vi "Supplementary Fig.10.vi"(3 "filepath":path) -> ()   [LabVIEW 2018]
uses:
  <vilib>/Utility/miscctls.llb/LVBoundsTypeDef.ctl
  <vilib>/Utility/file.llb/Read Delimited Spreadsheet (I64).vi
  <vilib>/Analysis/3filter.llb/Butterworth Filter (DBL).vi
  <vilib>/Analysis/NI_AALBase.lvlib
panel:
  out "current file index":i32
  in  "x":dbl
  out "output variable":dbl=68.582008670742
  in  "PCOcompressed":bool
  out "appended path":path=path "D:/大学/conference paper workshop/2018ViFFI/NCommn/reportchecklist/testimages.tif"
  out "size(s)":i32[](array[numeric])=[50, 88, 2560]
  in  "go":bool
  out "Array":path[](array[path])
  in  "review all files":bool
  out "img len 2":i32=70
  out "Boolean":bool=TRUE
  out "cs 3":dbl[](graph)=[22.65040892157367, 86.37730490337717, 155.79963793803236, 197.17804143502852, 212.85393455413336, 213.6452450101584, 210.82573019637186, 209.85631744380734, 208.5153495857973, 205.32869587141286, 202.08786171253874, 200.58274723476814, 201.02503833297055, 202.13900135116626, 202.65130109889043, 201.8843012705394, 200.89276924196565, 200.89702800042315, 201.32918494553184, 201.83283790754814, 202.84705166948518, 203.83063939953993, 203.44359282126754, 202.45792601226054, 202.63395668821033, 202.93321345821835, 203.15667855475328, 204.43918408682885, 205.67148460577496, 205.62475824945588, 205.46283059740284, 205.8138945597605, 205.80833242991133, 205.58843600987532, 204.60192113663442, 203.06170729060165, 202.23131126048585, 201.8641799176052, 201.30668848010538, 201.19635084533294, 201.96157151537406, 202.71980769348514, 203.27723713412033, 203.94056554984283, 204.18488561830355, 202.82728829485137, 201.36826216771493, 201.03099802192392, 200.7112090135604, 200.91265471875832, 201.30680696006576, 201.12311332384192, 201.40432765992006, 202.3164767282985, 202.39930349464566, 201.78281933763196, 202.24792538060763, 203.3800816469132, 203.31614273423315, 201.80453332483162, 200.49831835013848, 201.0398808130734, 202.0835068642121, 203.17981933909138, 205.62291661530793, 208.24427083572772, 211.36580763125718, 217.1450167772106, 226.14185557611017, 237.09115177491964, 246.07502920376032, 250.50482038078198, 254.51794286038157, 261.0230900964432, 269.72373715173757, 281.32337460851846, 292.9717516954466, 301.74712935377573, 308.96914350623297, 314.5127261014365, 315.7698306771272, 315.2048104451725, 316.4985840808151, 319.17590958776924, 320.2925476750582, 318.79315408433484, 319.15518315897964, 321.16787818269864, 322.6518956719798, 325.82091926094574, 331.1453319723793, 339.1117692119619, 344.0667454499893, 342.5681441424036, 343.2135713055129, 346.86002753615367, 351.44963207356125, 358.4665102360143, 359.9398685334197, 351.27714990813155, 334.9058862689725, 313.08353183385304, 303.43364672805143, 320.9407183868012, 342.12763830096344, 334.0072827765716, 298.20071977469155, 256.60459772605424, 223.36742331526776, 203.4557119569053, 196.15235288354899, 196.00154810766026, 197.8056656612016, 199.75213440726253, 201.7669588058611, 203.60351698833327, 203.29659749416388, 201.41873422982093, 200.72688499277828, 200.99345091694389, 202.06117453039934, 203.4671340637097, 204.4367775526614, 205.3704683880752, 205.2441285428637, 204.0327353325124, 203.2256293614327, 202.57558707235418, 202.03649450261787, 202.3307003542739, 202.29962244985785, 201.48883579279754, 201.2229334678881, 202.2188113001841, 204.41794090834088, 206.06170983615206, 205.41396074677795, 203.66954763507547, 202.92423305479753, 202.99827691279836, 202.73073788739418, 202.5514494622047, 202.862118680771, 203.0195210914974, 203.0643651013083, 203.63996340660358, 204.55821898163626, 204.45104395499254, 203.16523352272313, 202.1839469761759, 202.46843320863397, 203.55190028100589, 203.892787651315, 204.14591687422634, 204.75909563552855, 203.8859946870238, 202.07738571462303, 200.76087754519654, 201.29410427246535, 204.96934135088196]
  in  "low cutoff freq: fl 2":dbl=0.12500000000000006 format="%0.4f"
  in  "low cutoff freq: fl":dbl=0.12500000000000006 format="%0.4f"
  out "result":bool=TRUE
  out "x < y?":bool=TRUE
  in  "Threshold Limits 2":cluster{"Lower value":sgl, "Upper value":sgl}={"Lower value"=20.0, "Upper value"=60005.0} {"Upper value" format="%.2f"; "Lower value" format="%.2f"}
  in  "Threshold Limits":cluster{"Lower value":sgl, "Upper value":sgl}={"Lower value"=50.0, "Upper value"=60000.0} {"Upper value" format="%.2f"; "Lower value" format="%.2f"}
  in  "reverse v":bool
  in  "low limit":i32=81
  in  "up limit":i32=3
  in  "h/v align":bool=TRUE
  out "img len":i32=78
  in  "v cut param":T1={"thresh"=60.0, "ch1 back"=20.0, "img len"=70, "ch2 ofst"=68, "add ofst"=0, "debris size"=0.0}
  in  "h cut param":T1={"thresh"=1500.0, "ch1 back"=7.0, "img len"=78, "ch2 ofst"=70, "add ofst"=0, "debris size"=15.0}
  out "cs 2":dbl[][](graph)
  in  "thresh2":dbl=1000.0
  out "xy shift":i32[](array[numeric])=[-1, 2]
  in  "y shift":dbl=2.0
  in  "intervals":i32=40
  out "Histogram":T2(graph)={"X Values"=[4559.940789473683, 4813.127631578946, 5066.31447368421, 5319.501315789473, 5572.688157894736, 5825.874999999999, 6079.061842105262, 6332.248684210525, 6585.435526315789, 6838.622368421052, 7091.809210526315, 7344.996052631578, 7598.182894736841, 7851.369736842104, 8104.556578947368, 8357.74342105263, 8610.930263157894, 8864.117105263158, 9117.303947368422, 9370.490789473686, 9623.67763157895, 9876.864473684214, 10130.051315789478, 10383.238157894742, 10636.425000000007, 10889.61184210527, 11142.798684210535, 11395.985526315799, 11649.172368421063, 11902.359210526327, 12155.546052631591, 12408.732894736855, 12661.91973684212, 12915.106578947383, 13168.293421052647, 13421.480263157911, 13674.667105263175, 13927.85394736844, 14181.040789473704, 14434.227631578968], "Histogram: h(x)"=[13, 6, 12, 7, 11, 10, 12, 18, 10, 17, 8, 14, 12, 14, 15, 16, 28, 30, 21, 12, 10, 11, 4, 5, 5, 7, 7, 8, 6, 2, 5, 10, 4, 4, 6, 5, 3, 3, 1, 2]}
  out "cs":dbl[][](graph)
  in  "skip failed img":bool
  in  "decline thresh":dbl=20.0
  in  "color 1":T3={"color array"=[0, 65280, 16776960, 16448250, 65280, 16776960, 16711680, 16448250, 16448250], "num of colors"=4, "max"=24.0, "min"=0.0} {"min" step=0.01 format="%_2f"; "max" step=0.1 format="%_3f"}
  in  "mgn":i32[](array[numeric])=[10, 10, 10, 10]
  in  "iter":i32=10
  in  "input 2":T4={"Niblack Dev Fac"=0.6000000000000001, "Window"={"Width"=50, "Height"=50}, "Sauvola Dev Rng"=2.0, "adaptive"=FALSE, "Method (Niblack)"=1} {"Method (Niblack)" items=["Niblack", "Background Correction", "Sauvola"]}
  in  "in1":T4={"Niblack Dev Fac"=0.5, "Window"={"Width"=20, "Height"=20}, "Sauvola Dev Rng"=6000.0, "adaptive"=FALSE, "Method (Niblack)"=0} {"Method (Niblack)" items=["Niblack", "Background Correction", "Sauvola"]}
  in  "post proc 2":T5={"trunc for ch2 masking"=[2, 2, 5, 2], "Erosion(pre)"=2, "Op"=enum."PClose", "post proc"=TRUE, "move x/y"=[0, 0], "conv"=FALSE, "Conn"=TRUE, "iterations"=5, "Erosion(post)"=2}
  in  "post proc1":T6={"trunc for ch2 masking"=[0, 0, 0, 0], "Erosion(pre)"=2, "Op"=enum."PClose", "post proc"=TRUE, "move x/y"=[0, 0], "conv"=TRUE, "Conn"=TRUE, "iteration"=5, "Erosion(post)"=2}
  in  "seg meth 2":T7={"norm for thresh"=TRUE, "use thresh formula"=FALSE, "thresh"=0.27000000000000013, "man thresh"=FALSE, "Meth"=0, "upper lim"=65000} {"Meth" items=["clustering", "entropy", "metric", "moments", "inter-class variance"]; "thresh" format="%_3g"}
  in  "seg meth":T7={"norm for thresh"=TRUE, "use thresh formula"=FALSE, "thresh"=3.378, "man thresh"=FALSE, "Meth"=0, "upper lim"=64100} {"Meth" items=["clustering", "entropy", "metric", "moments", "inter-class variance"]; "thresh" format="%_3g"}
  out "mask2":u8[][](graph)
  in  "lpf 2":cluster{"cut":dbl, "lpf":bool, "odr":i32}={"cut"=0.2900001, "lpf"=FALSE, "odr"=2} {"cut" min=1e-07 max=0.4999 step=0.01 format="%_2g"}
  in  "bg calc rng":dbl[](array[numeric])=[0.4, 0.6]
  in  "bg":u16(ring)=2 items=["calc bg", "load bg", "no bg correction"]
  out "cells":i32
  out "x = y?":bool
  in  "lpf 1":cluster{"cut":dbl, "lpf":bool, "odr":i32}={"cut"=0.15000010000000014, "lpf"=FALSE, "odr"=2} {"cut" min=1e-07 max=0.4999 step=0.01 format="%_2g"}
  out "mask1":u8[][](graph)
  in  "idx2":i32
  in  "show imgs":bool=TRUE
  out "N of success":u16=10
  in  "bg filepath":path
  in  "search subholder":bool
  in  "save img":bool
  in  "mask img":bool=TRUE
  in  "sec unit":i32=300
  in  "scale fac1":dbl=1.0000000000000009 min=0.01 max=10.0 step=0.01 format="%_3g"
  in  "scale fac2":dbl=0.9999999999999983 min=0.01 max=10.0 step=0.01 format="%_3g"
  in  "autoscale":bool=TRUE
  out "ch2":picture
  out "ch1":picture
  in  "color":T8(array[cluster])=[{"color array"=[0, 16711680, 16776960, 16448250, 65280, 16776960, 16711680, 16448250, 16448250], "num of colors"=2, "max"=4900.0, "min"=0.0}, {"color array"=[0, 65280, 16776960, 16448250, 65280, 16776960, 16711680, 16448250, 16448250], "num of colors"=2, "max"=9000.0, "min"=0.0}, {"color array"=[0, 255, 16448250, 16448250, 16776960, 16711680, 16448250, 16448250], "num of colors"=2, "max"=1.0, "min"=0.0}] {"min" step=0.01 format="%_2f"; "max" step=0.1 format="%_3f"}
  in  "unmix":T9={"c1 -> c2, c1 <- c2"=[0.03, 0.02000000000000004], "unmix"=FALSE}
  in  "image lpf":cluster{"cut":dbl, "lpf":bool, "odr":i32}={"cut"=0.2500001000000001, "lpf"=FALSE, "odr"=2} {"cut" min=1e-07 max=0.4999 step=0.01 format="%_2g"}
  in  "reverse h":bool
  out "mixed":picture
  out "curr img size":i32[](array[numeric])=[2560, 88]
  out "curr index":i32=1311
  in  "review all imgs":bool
  out "num of files":i32=50
  out "max2":dbl=17870.242105263158
  out "max1":dbl=14560.82105263158
  in  "file type":string=".tif"
  in  "frame index":i32 min=0 max=49
  in  "transpose":bool=TRUE
  in  "Draw Area Size":T10
  out "max value":dbl=24.0
  in  "autoscale":bool=TRUE
  in  "zoom 2":dbl=0.5000000000000014 format="%_2g"
  in  "frame [ms]":u32
  out "cycle time":u32=17
  in  "zoom":dbl=1.9999999999999973 format="%_2g"
  out "entire img":dbl[][](graph)
  out "x proj":dbl[](graph)=[-0.6834175105647228, -2.7922158127679118, -6.30996339498379, -10.48569202110438, -13.54291741641208, -14.349970108657555, -13.701267260419232, -13.894588588034273, -14.878874404013395, -14.863747871840786, -15.302439752050166, -16.30687103819798, -15.643161215622314, -14.487337019319579, -14.595162853469436, -14.593941392233873, -14.166323551069151, -14.251724102511528, -14.572410867893547, -15.041552545206267, -15.572230117774634, -15.818546099314855, -15.190464999042959, -14.320936985804096, -14.686809209149082, -15.419230593399906, -15.20675810543543, -13.981248077775604, -11.920339576425084, -10.971586187658659, -11.25221777963731, -11.344895546808072, -12.022146630222142, -13.117927850718345, -14.413445296549057, -15.269610451173484, -14.961554040865941, -14.580989432911498, -14.81303051441752, -15.451549032211478, -15.195154453333984, -14.838214893162156, -16.149251075164745, -16.918501257161715, -16.132803421003587, -15.52614796154118, -15.508980206767735, -15.695012778831137, -15.876128554725758, -16.18013743433353, -16.89454319413985, -17.46675511064096, -16.694164623634443, -14.993973438041495, -13.648547978181846, -12.653905866235657, -12.45751666205452, -13.775479390585971, -15.669316073200875, -16.82025936546387, -16.200158411236686, -13.572145620867065, -11.203500645851197, -11.017897885818662, -11.632458250522696, -11.980845686827687, -12.885503640350821, -14.208080630663469, -15.543989815895518, -16.460269150631753, -16.0001628738515, -15.358575144040161, -15.492835627959574, -15.540386983916306, -15.052309972922913, -14.088140737295321, -13.341805601328163, -13.447699196986228, -14.186839306825282, -14.653147274282508, -14.45588231379865, -14.11446313631473, -14.639373619143873, -16.322012163187026, -17.538186689406707, -16.952354638933542, -15.115955719718634, -15.92300531539663, -20.713119497102248, -23.007644467175748, -20.547675366789306, -17.36592152730349, -14.893231720663183, -13.13438666240775, -11.909837282538096, -10.365292012040246, -9.610157111318731, -10.877523616870858, -13.202799507317867, -15.167897285029014, -15.659730836338658, -14.784985852331703, -13.893954928165991, -14.028882088433711, -14.35547187020653, -13.739728292820661, -13.24559856604987, -13.277869669877969, -12.691956483769992, -11.640639835026786, -11.040015534270898, -11.507597906403465, -12.636802259475491, -13.545565542634765, -13.830692185755483, -13.60132892262358, -13.87582738758939, -14.796867880930424, -15.08557833270453, -14.757870440442604, -14.84082302405131, -15.321160652800952, -15.941638596870938, -16.07362505091237, -15.40545065416542, -14.438601088064821, -12.871091717770776, -11.520250753517509, -11.452586312676168, -12.620120570977653, -14.622116896115239, -15.632283681879436, -15.136297369122076, -14.33195472703209, -14.03183520127222, -14.016994012860485, -13.61488608346895, -13.14309108181286, -12.441790173190853, -12.035493409162154, -12.764879772451389, -13.197459793492103, -12.87401599608488, -13.303556575539167, -13.42582162495954, -12.519234369430755, -12.892944639653322, -14.230895323758885, -15.270126162912508, -15.803938832988939, -15.179763381627646, -14.315716492920693, -14.490192341186564, -15.333229669789583, -15.874632123623439, -16.10405880936504, -15.456479367886422, -14.086042542839127, -13.888521783534085, -13.475692190212179, -11.297322584278787, -9.771670180089135, -10.719122741028414, -12.901988966851139, -14.93709067962128, -16.42107411849932, -15.970247009387723, -13.976600186118329, -13.028296221958328, -12.994037757345598, -12.78968452385558, -13.09659330053799, -14.039853852258632, -14.826865503427738, -14.961553801260065, -14.338046564506225, -13.119515767298509, -12.666665024518577, -13.62220091151925, -14.283514741181664, -14.19797114502582, -14.58029943646456, -14.676383319724124, -13.370325361607014, -12.30219629465311, -12.413924716022782, -12.582413085396315, -12.996915855133329, -14.014967534975739, -14.54373505480318, -14.995804512257399, -15.636288135977123, -15.210772411813558, -14.107942433807814, -13.014760788061801, -12.742233532780755, -14.411783421344659, -16.3695857888955, -17.463640787256267, -17.940156015453052, -17.438947443968026, -16.807565061654586, -15.110157618550565, -11.670034796353715, -9.87113803290875, -11.6649752573667, -14.541639903820691, -16.07005316298409, -16.16164249576132, -15.543260514552726, -14.734452468049788, -13.885135037158573, -13.842148930997821, -14.865775635246669, -16.43097528689782, -16.784402185436797, -14.838523730819883, -12.690860817932032, -11.509913102805502, -11.600547921666902, -12.763065997311815, -13.828886943745289, -14.641508689410983, -14.759488950986187, -14.697478966043427, -15.380737221215163, -15.752696058094127, -15.192211950311329, -13.85637867630627, -12.5885088775801, -13.986311130425905, -17.484154311875482, -19.046814456908745, -18.280215041100195, -17.622357903220184, -17.06239523828483, -15.77743235808388, -15.143136249929485, -15.07106817712601, -14.335874126088605, -13.862011364263319, -14.44136253512707, -14.462116800645607, -13.214625250557301, -11.93392977639283, -11.337571166409074, -12.080897024719594, -13.761546151606957, -15.586457422748946, -17.03967711245096, -17.21569558063286, -16.018561164245824, -14.928850262697573, -14.983923288034408, -14.813297163825101, -14.145916271389098, -14.647520708873756, -16.123946788813186, -17.25110209410827, -17.82165228056119, -17.983853719926973, -18.04422638097217, -18.24234127109032, -17.530321903976997, -15.230888143169889, -12.616883481434947, -12.090427047136432, -14.027511215130799, -16.029297161120862, -16.6851178900205, -15.855121037384794, -14.072937007099437, -12.864605553004116, -13.002858586848216, -13.731244094423328, -14.17662604623215, -14.64663422697672, -15.527087976424205, -15.517100827951875, -13.94499632273175, -12.466131030389096, -12.865082244751546, -14.710482883628332, -16.024466334368416, -16.160012901234012, -14.873502217072105, -12.736706466556772, -12.615419101744688, -14.677799621809232, -15.783980088472472, -15.553650423082287, -15.553553147413675, -15.434975844288209, -14.346901786619798, -12.970057203096355, -12.620433471080204, -13.726063979269703, -15.177896881858572, -15.8852613477424, -16.26348880688422, -16.28666584690531, -15.20613082070219, -13.98440480236911, -14.6571949020836, -16.675060226670517, -17.572209949311954, -17.06201153404411, -16.672466239332874, -16.18237233298253, -14.580951850229942, -12.746327410477114, -12.038589093044003, -13.25207243640323, -15.217854714436147, -15.788037915720603, -14.986933523340761, -14.041583991859127, -14.003121141209725, -14.965392038911046, -15.202033181366888, -13.932810748930311, -12.5596649100939, -11.590493669035851, -11.13446553973715, -12.00388590594944, -13.756641248085415, -14.240668387154688, -12.74592674839886, -11.565852728612187, -11.830195142380187, -12.863301858501114, -13.846841146394226, -14.527393047335213, -16.01274997876434, -17.186307290045313, -16.33316266272545, -14.747100132132857, -13.438496507277772, -12.24526532342578, -11.654108455815297, -11.00634877930038, -9.8116388052108, -9.68222391524505, -10.934757774278028, -12.451689536930694, -13.75724845069177, -14.775390496833003, -15.39774879190061, -15.449870991671233, -14.803404143170503, -13.297855630290385, -10.922326954053016, -8.501089033287602, -7.205429067723376, -8.06015239248695, -10.664714947442652, -13.323567663388861, -15.450325890588493, -16.373906391926973, -15.266543081959618, -13.71938862801769, -13.117993888128822, -12.871449495240045, -12.058421542266892, -10.88591753675202, -11.223052351972944, -13.200944720691913, -14.953341257456014, -14.87227729819865, -13.625930847916097, -13.356565121838807, -14.591995298877666, -16.822869344770503, -18.31908536098044, -18.205058083756246, -17.69644453667013, -17.15729710527646, -16.135104370676746, -14.081883680529572, -11.998664196339602, -11.597672584201458, -11.816389488471224, -11.668106269387222, -12.138815385528066, -13.998866957004868, -16.279054868253226, -17.6135573111164, -17.818782424364908, -17.17691207732298, -15.91755610189869, -15.237073902859034, -16.479760552177495, -18.26872845243941, -18.271950732608648, -16.116568927060992, -13.692857087588177, -12.809637763557653, -13.468252056217336, -14.676499226409021, -15.010321047751553, -14.336515784833214, -13.492341077302898, -12.921047284674534, -12.956711119575031, -12.985504423910527, -13.098394139546045, -13.195229816037006, -12.760742097479472, -12.611717807950198, -12.713676672823652, -12.761848102734396, -13.066171492922482, -14.215712849893492, -15.686225069544669, -15.517883958411224, -13.599795748689289, -11.749887472784824, -10.938033179552045, -11.667925359853475, -13.798265279819777, -15.563471624573406, -16.12708652825845, -16.26532778638087, -15.817266968145418, -14.958226466408965, -15.273979649743305, -16.24854573156266, -16.378706873444983, -16.078937541330014, -15.948187403204532, -15.729575955621078, -15.469419412683399, -15.589905173116293, -15.497325866266758, -14.100675390369688, -13.01002260858952, -14.009392630337985, -15.608051868802011, -16.196372475024862, -15.437111465596924, -14.329904306370954, -13.831999607704418, -13.829270681968556, -14.773714642502364, -15.762685662610984, -15.696864318156036, -15.988567863336673, -17.06657763484871, -17.1070208228435, -15.711872633335386, -14.968819680882266, -14.53804988956229, -12.915134458882505, -11.626256120492368, -11.537848217412378, -12.17701577865142, -13.394884473127112, -14.622939454805643, -14.691387053035436, -13.370257677583378, -12.590024455920004, -13.368731780793084, -14.5582439738597, -14.443846986885811, -13.060808752441186, -12.966573004398207, -15.193729819736445, -17.22729424533496, -16.742443327373227, -14.924049179001983, -13.078374488598115, -11.944387085456592, -12.662051280789695, -14.497715957519178, -15.891544740670364, -16.007984456639228, -15.457893133394554, -15.486235259114254, -15.891582391790967, -16.0690378123424, -16.198859749361624, -16.066843092652928, -14.825160813746137, -12.722186357278648, -11.543901410225176, -11.036364121134463, -10.560090733306247, -11.93996321330335, -14.571250134871434, -15.322889793998462, -14.373398236609846, -15.277914990049853, -17.814033770381194, -18.14624458964294, -16.344879078785553, -14.633429521139025, -14.30373208482877, -15.149159984398118, -14.884563322300771, -13.962765605295242, -13.962933854061045, -13.098785510933382, -10.917167535713078, -9.538892122857916, -9.84532725000828, -10.984186487913647, -12.443923596805718, -13.733450414247018, -13.77923141023114, -12.611503291194628, -11.300036184587048, -10.940971209774544, -11.625383644835313, -12.976128639346207, -13.728592535875752, -14.280667188297699, -15.721919738640011, -16.018041133724946, -15.035760962133606, -14.596737640922434, -15.486559937461113, -16.66709569698512, -15.628517666977206, -13.279514260677752, -12.582618162434674, -13.587259011841349, -14.571480041743369, -14.774007952763377, -14.832141567687396, -14.62417901590864, -14.115838951326356, -14.779833995148683, -16.649243016540137, -18.28803813598679, -18.136030849121834, -15.493830506107296, -11.97946742634762, -10.132614024646431, -10.83204224715748, -13.083398029223806, -15.070484948474796, -15.900583316185184, -16.606631693874956, -16.89796995931394, -16.058617194458368, -15.658310428218389, -16.048837209241803, -16.6480960510551, -17.375800330503644, -17.764502484556782, -18.278930588482257, -18.243846379671464, -16.672457614616626, -15.495526034166168, -15.886011283190463, -16.25595054164054, -15.986415504979586, -15.511351276304644, -15.055670365460198, -14.979667171406987, -14.7670110909992, -14.396589267785435, -14.41113080260957, -15.231732144756222, -17.26975927958338, -18.917695908572455, -18.034683771181193, -14.993131494616081, -12.810390178707678, -13.816585221183711, -16.273864026963835, -17.47416177174676, -16.908040746418262, -15.778935330972239, -14.805480471895468, -13.77591153631215, -13.422602806751218, -13.237427641370106, -12.301932741252294, -12.16508225675907, -13.617093964198205, -15.32457377743269, -15.669348697686765, -14.644197088565672, -14.148536346702784, -14.70635763132227, -15.202234683460434, -14.995656258833773, -14.147444536898169, -13.709495549970399, -13.872223744801845, -13.585841916224943, -13.359226880225172, -14.510236733043408, -16.256744012190637, -16.836279404655404, -16.800501519538916, -16.768853487683117, -16.262786034117607, -15.405686115446294, -14.278138349083143, -13.500776093030744, -13.827138695459016, -14.589219205755747, -14.515510556569495, -13.899097320094867, -13.63540011593793, -13.982779378195001, -14.788715047312664, -15.23750324979562, -15.391979601812698, -15.680918454524143, -15.804209427048, -15.824136319785122, -15.216040145960125, -13.85503069404488, -12.969819547584507, -13.174690729924428, -13.858177661023209, -15.020071362979913, -16.66873485701156, -16.664238929804828, -15.036503828657484, -14.577300902713514, -15.663249328639887, -16.44963467352514, -16.340907713519364, -15.390484066640202, -13.651978722590698, -11.939183755923876, -11.880157685702155, -13.85990512263093, -15.160317825329965, -14.750132137535013, -13.44177909676561, -12.14971843706951, -11.953456082718917, -11.90621182826691, -12.024721375728102, -13.323774208659461, -14.801923001366326, -15.860148509894666, -16.560398969007977, -16.67259745118025, -16.349700229043975, -16.20313246033038, -16.07494837722363, -16.19821333346385, -17.33346740579777, -17.386396161562132, -15.886306971691344, -15.528308204029525, -16.08133775071093, -15.15997476313304, -13.521175788011508, -14.919261262111878, -18.44338345298166, -19.054414549237087, -16.698433481637196, -14.566409416036164, -13.927431310277164, -14.32856488214173, -14.72448779662178, -15.354580601292845, -17.085867437937466, -18.898633677958944, -19.05431973773286, -16.937118309252604, -13.61990235818136, -11.686290340813652, -12.14057497353854, -12.72526060715683, -12.344030714604456, -12.473126024343344, -13.307701318068705, -14.344407899774469, -15.141263546836994, -14.375404519900869, -12.509047499267052, -11.688133078270088, -11.82917976548044, -12.528691216613334, -14.11749210440634, -15.382257462980228, -15.166409726152107, -13.565007346029395, -11.24846029200768, -9.402937431724318, -9.11856165450807, -10.246672470805326, -11.990843911682553, -13.259227577445067, -14.068942831304195, -14.89771050318441, -14.725757562419561, -13.701596446886196, -13.67200539048654, -15.938115172230452, -18.475011940893992, -18.158829765945974, -16.52694273170763, -15.777196449867914, -14.930873710638284, -13.601819823773459, -12.82614552810636, -12.928375042868169, -13.673840344009115, -14.733119556941165, -14.409387340423788, -12.286610514595193, -10.783672360533515, -11.1482227575377, -12.285796771446254, -13.334426111164465, -14.04152306888732, -13.968113068912926, -13.565571398349089, -13.698676836408511, -14.739398987251828, -15.96912598030195, -15.610043449158876, -14.178170683874919, -13.436037636106873, -13.116007737437805, -13.549813702674452, -14.260748667757124, -14.005374008899139, -14.01578151453176, -14.598874055917594, -14.168839078092839, -12.88561652177645, -12.893069488243555, -14.20651672096117, -14.954206960763488, -14.635533897285665, -13.69533168004474, -12.426969518518016, -11.349284797834724, -11.244176651064338, -11.992463344862138, -13.709301583771888, -16.0548340297954, -17.010526303695826, -16.446299961260035, -15.40051602693702, -14.212092633843344, -13.440230958381331, -13.694440360563197, -14.972447092051977, -15.79973370749493, -15.079762962368783, -13.929943683165988, -13.866922502426146, -14.483671875294496, -14.59800045598237, -14.109683059525423, -14.001707767839312, -14.64846658968274, -14.513179835032515, -12.803208964464737, -11.333759624672707, -11.20175730172397, -11.762382910611045, -12.725470869679743, -13.837127994117441, -14.2712858436734, -13.138488539642207, -11.632864497123043, -12.153044804961448, -13.731136620911064, -13.971640615172891, -13.47709720430737, -13.223562425814698, -13.051744274980328, -13.071895234634479, -13.441059677351213, -14.270549629912857, -14.734283296974901, -14.406843575624034, -14.13881470261628, -13.799999085647505, -12.886486105644666, -11.942894201609375, -11.162509403713246, -10.546024049146379, -10.420186494698825, -10.60467190172187, -11.308707627674748, -12.594401250590288, -14.060041612350918, -15.40382034790587, -15.986938156543614, -15.600625288960723, -14.74914020283138, -13.879861174841682, -12.855970044949355, -11.301716249647402, -10.275279834758745, -10.899572702942617, -12.02556928116676, -12.586178194365536, -12.641762080841636, -12.507297433844652, -12.850150351413143, -13.315847803966317, -13.445365121143386, -13.607504880510621, -14.01009249139642, -15.11665772801527, -16.22100371378028, -15.819394213005449, -14.291589232398803, -12.887399643562539, -12.365678548794644, -12.146596233866502, -11.723426186339548, -11.788009369465076, -12.575742098585861, -13.980313420807267, -14.94434731363307, -15.092163524626866, -15.20307457271574, -15.258370441334009, -15.078271390990851, -14.499516129989622, -13.623369162084257, -12.794986153446477, -12.208397079373798, -12.614900776755476, -14.36525870469483, -16.075272898575975, -16.908774953278694, -17.710389932962833, -17.5049082548777, -15.579507183604274, -13.83271553763094, -12.437100645387138, -11.215410823715128, -10.724057723790883, -10.570404446192448, -10.686954186383158, -10.945687167366295, -11.443666266609224, -12.998494012153783, -14.78656200036396, -15.27067524086572, -14.350030334921108, -12.734880475715897, -11.909508512013375, -12.548403304808385, -13.621145225851697, -13.73615356679905, -12.51069310077562, -11.121719633782611, -10.80645615021873, -11.362738334849654, -11.699400817231883, -12.319537219395425, -13.57303518241118, -13.962345823865713, -13.325772324647668, -13.083990224824273, -14.04453777080227, -14.542589350605166, -13.910925784389027, -13.93041905315739, -15.233293807590229, -18.50541068155657, -21.741886908261225, -21.26178350956289, -18.461108327282645, -16.078271982064933, -14.277115360587644, -12.396936664914513, -11.322303804274165, -12.205060406963916, -12.809755829415959, -12.499829502583541, -13.56816018560935, -14.581069715638614, -13.617842584174491, -11.493387169082851, -9.616244959908883, -9.140396555421791, -9.024583228160164, -8.781116292097778, -9.664119708188412, -10.870672176794095, -11.713886281308476, -13.278264882086075, -15.25315238668777, -15.324430700349527, -12.78071524531497, -10.35871787720911, -9.801821667989485, -10.084107342749734, -9.364308023708855, -8.103424127983331, -9.009574882873586, -11.358138441845028, -12.098762273089559, -11.330757087376178, -11.336110973267026, -12.475840050303999, -13.2557090816447, -12.732387306856545, -11.39325202452236, -10.305143764032195, -10.018537104080119, -10.79444201776111, -11.91440095791831, -11.73536267229401, -10.31456445465864, -9.034702477349768, -8.204005366106507, -8.237961569664487, -9.523185551856013, -11.114111899956233, -12.771430088999317, -14.291811244396557, -14.68464558331928, -14.157695339682519, -13.23704388706355, -12.642326527538795, -12.876660806021794, -12.80767703768067, -12.176371726316166, -11.604165960209976, -10.786964929378746, -10.20723566408961, -10.811741671156058, -11.574918488738684, -11.800053271512475, -11.855551180696493, -12.32098554836191, -13.619981631838915, -14.884804240974551, -15.741922811310529, -14.956841537498823, -13.052273967620033, -12.299372783874109, -12.126755524109058, -12.410239617993726, -13.516098654943779, -14.464217855733967, -15.380017823504435, -16.317926871553535, -15.432463252245098, -13.308693067241252, -12.675479676662686, -13.665083418216021, -14.223375465901892, -13.150666394260757, -12.050840306239586, -12.543056892086254, -13.17846968977057, -13.222946133530801, -13.834123244453131, -14.590783215260934, -14.41702586293625, -13.122306213413552, -11.178503355468614, -9.582179516577003, -9.799027056274646, -11.609522625959602, -13.048929559694665, -13.509623689294225, -13.268905822963811, -13.08365227812627, -13.477388214534201, -13.812726124050073, -14.192902570866526, -15.415867788527835, -16.53979604394496, -16.0202178174342, -13.984139140611163, -11.944805278086763, -11.188951130657719, -11.839520471083837, -13.1929898745791, -13.373516962450047, -11.920990190059694, -10.686621265828707, -10.007022674212594, -9.09432977490276, -8.753260739931191, -9.907501611646746, -11.988099676427948, -13.272066167749838, -12.715126894280122, -11.957312827075732, -12.502427099483256, -13.171339380334809, -13.229766877526488, -13.257144235747598, -13.654004315967132, -14.019041801767395, -13.840391458738482, -13.647910211053484, -13.330725118868406, -12.90057841612064, -13.479440236065384, -14.754365065612097, -15.470528563451174, -15.623127968344837, -15.137754609320996, -14.43401160371674, -14.420462819446609, -14.739900977940186, -14.947955350479816, -15.037631507886339, -14.564672177701244, -13.79597657361985, -14.107576174369582, -15.341004473901641, -16.302394220322597, -15.723716596905879, -14.076622269077852, -13.888192260855774, -14.942987698572681, -14.731064428820757, -12.227041315981689, -10.132128920659497, -10.944322402730103, -12.310738819976537, -12.742490974405536, -13.182234034930673, -13.452910383557073, -13.171001180458148, -12.326833820640067, -11.62491493556143, -11.439790730067081, -11.499226917004197, -12.007496251695056, -12.173991894874673, -11.28286272464446, -10.191937392131718, -9.16755296287774, -8.467764765487638, -8.83287711277855, -9.605633213336676, -10.798276973743842, -13.03196194871889, -14.545090273160012, -14.250808950813825, -13.761874970003525, -13.984783803901166, -13.674504750987088, -12.526619326351087, -12.3288575037779, -13.013189708943907, -12.943256323442064, -12.844473906102783, -14.043856026578217, -14.81704751476948, -14.365176817049477, -14.169573906238394, -14.23341235221042, -14.65169400535721, -15.122405320819038, -14.352827184979844, -12.98220282379709, -11.946491828741078, -11.133995706383782, -11.10372830607823, -12.029441478755459, -12.814670288364535, -12.367740395775261, -11.684627915552433, -11.775346361270799, -11.698056400455352, -11.497316171731086, -11.236188716414595, -10.568753435422558, -10.80758048644044, -12.426800091765632, -14.361961323656292, -15.744340034497975, -16.012081146255248, -15.510823764795893, -14.85135566320602, -14.20142682233628, -13.515597516495845, -13.183265465861929, -13.68433600995715, -14.365158272549689, -14.449495850982615, -14.497331474152436, -14.319056660166714, -13.256352689490981, -12.606743934221438, -12.44615265609217, -11.632602342388832, -11.212003395703942, -12.160584146106642, -13.390376449027604, -14.62416645977322, -16.158512653180033, -16.412796196823255, -14.481360049817107, -12.087468041277797, -10.474297060057935, -9.751348876192479, -10.29088796282014, -11.040553019934777, -11.274604432917918, -11.538275087715387, -12.00174224621071, -12.643706274264076, -12.606311346762372, -12.161804915777699, -12.829127011753872, -15.168550294821006, -17.83515653009029, -18.690769581578547, -17.046483390522447, -13.356040766331608, -10.815277781574618, -11.89548568599545, -13.956098605866455, -14.757745212945501, -14.924304981900693, -14.716492429404633, -13.488734223593863, -11.619414953608375, -10.852043017159641, -11.142188532299201, -11.57389991989236, -12.567623658320665, -13.262980514943395, -13.19680370859935, -13.390781363050003, -14.572034914357149, -16.206858662407132, -16.57338550619015, -15.983484787390047, -15.402776514413032, -15.051913077062165, -15.305209572044149, -15.465712130955527, -15.044447865011149, -14.984299544964172, -15.263274732845003, -14.47240270005577, -13.438507521638453, -14.094200831437695, -15.740443649125117, -16.585816460991513, -15.662521110377188, -13.43629716616253, -12.328575730406634, -13.002591322671435, -13.22625121230874, -12.529030403845049, -12.968703900354367, -14.787211859615727, -15.183586898372699, -13.48665745494916, -12.242807384532732, -12.612048168957653, -13.374788409173135, -13.97082654255179, -14.864316374717294, -15.80092050806514, -15.995605117562182, -14.695381274616441, -12.818837171947369, -12.264070956174587, -12.659440271682886, -12.338440452592124, -11.51348485721978, -11.623757786198478, -12.197971445014415, -12.214432266664012, -12.917226781648836, -14.941175885330384, -16.51747748871717, -16.157406316169542, -14.413814434842632, -12.88996396848108, -11.839199118676369, -10.282536870841728, -8.969894432953037, -9.129890346532497, -10.30406985739453, -10.088560997290877, -8.224780176965137, -7.808631002927639, -8.52569743712918, -9.633363764868689, -11.317339105424008, -12.340522027178661, -12.353338731731588, -11.92673038981134, -12.203665463548345, -12.606965135638873, -12.016208365266875, -11.81295968144325, -12.794564637480189, -15.154615247697567, -18.41932567071891, -19.734329909573326, -18.90958025863206, -17.986557303211626, -16.414928736189026, -13.678760264659855, -11.525321006480095, -10.992881598173739, -10.818181704236554, -9.561748919246305, -8.8259303191477, -10.113101985345642, -11.864825155818297, -13.184939450160552, -13.552754200483818, -12.48318444522358, -11.44981056552491, -11.417846017790584, -11.341643221324869, -10.694666947441025, -10.891141382392043, -12.463610889318682, -14.075920025619835, -15.169494227778864, -15.663089494448236, -15.080513330128499, -13.390412770063019, -11.503007370934535, -10.67743564061183, -11.211631792396581, -13.162040206305637, -15.994410385042386, -17.428872023066205, -15.786919500591262, -13.077300426647412, -12.046275301359756, -11.977421849121562, -14.892220202890876, -20.98272607584496, -23.410164878910667, -20.7396753178756, -16.729349836027936, -14.32669726375579, -14.374540584831275, -15.122900818340119, -15.421989547409622, -14.575840037801667, -12.897337803087348, -12.2802980669837, -12.550941388487995, -12.914155198142778, -13.849799531976064, -14.610862199734187, -14.82125537362038, -15.156452696079324, -15.304717631507835, -14.649353201795044, -13.78678590091208, -13.387266606446483, -12.614701126400764, -12.01949250475467, -12.496894844823583, -12.36434837789248, -11.299199673581235, -10.339150000170875, -9.593793909939794, -10.28502380899112, -13.430688315275397, -16.361301433109183, -16.220764756735257, -14.427976957733367, -13.467983480552416, -13.746275321033943, -14.035755991351973, -13.727761673174783, -13.73141258022002, -12.958839804677618, -10.569505997658114, -9.160131177183473, -10.092270549868978, -12.026678022903294, -13.832634973168908, -14.49998073182459, -13.257970748666441, -11.57165070177774, -11.274455898729723, -12.825568581792716, -14.972823015873363, -14.918139182875695, -12.002947688038262, -8.686920295468049, -7.703843061152014, -9.932583951949606, -12.849708791265005, -13.880776105551147, -13.587607526687938, -12.576992143314625, -12.50294626543195, -14.234473030797316, -14.817712277903357, -13.130691685082429, -11.345740334467045, -11.299154062245716, -12.43600232474721, -13.42573083000977, -14.175168538524614, -14.551835684460766, -14.559517232873514, -14.63646589673399, -14.70645327662172, -14.453895237742902, -14.485345327347925, -15.575493498523887, -16.7880738336467, -16.689243157079414, -15.313191600144808, -14.048781309439551, -13.315367707404764, -12.264320245586308, -11.420223323192438, -11.951060996105562, -12.732905194538397, -12.316778353580135, -12.93303942086039, -15.312493113996211, -15.788346047145328, -13.784105023993487, -11.931132967348846, -10.754583426658161, -9.481930650538102, -8.674245286647826, -8.53223196073423, -8.66756896766784, -9.330659061459125, -10.398869426313595, -11.868375295911028, -13.190661813620695, -13.361703770586715, -13.179832574472094, -14.122921655970357, -15.072698301062449, -15.263268990621395, -15.02871747182958, -14.158270178382633, -14.001574877124392, -15.120300957518523, -16.32490886119167, -15.916142515617405, -14.250538284784126, -13.597495588284467, -13.732264585638854, -12.319647600822021, -9.868954733810195, -9.88428205474159, -12.375358653779111, -14.32833479589678, -14.362948764955359, -13.646960007638455, -12.862750270944963, -11.776266722172377, -11.892003110864275, -12.949068045114153, -13.22368211586893, -13.130235766638899, -13.341119971848332, -13.571092290323312, -13.131831098798397, -11.859985652818395, -11.29545402871754, -11.870574501814303, -12.600980491882503, -13.781324549543633, -14.943588154741594, -14.962515260638897, -13.518996903161211, -12.151725708742456, -12.613026798367272, -14.089489138990361, -15.132482007534652, -14.744991344322433, -13.934366281064744, -14.373206998812428, -15.252420495614174, -15.544546398879342, -15.624525249095306, -15.212030439374594, -14.01541840292304, -13.220002171473128, -13.259471527209476, -13.56182233647976, -13.443200669526052, -12.64479304867756, -11.736325534649179, -11.73173645968271, -13.006543072366126, -14.209971964728146, -14.23622255722228, -13.566935670238514, -12.927175744279861, -12.449468857700943, -12.505229013274658, -13.498084404471761, -14.220308579875681, -13.008179098424861, -11.429368926067909, -11.711730602241094, -12.016058436296666, -10.939656962933324, -10.311528674811338, -10.956803793057944, -11.384026813138167, -11.083569468470508, -11.243674331574933, -12.763979040525221, -15.022647434822222, -16.157216817895225, -16.0834853340417, -15.14762546536858, -13.508816897311728, -12.3733177244211, -12.825339089574651, -14.508688300366924, -16.140353513933025, -17.117585826520646, -16.421099079716377, -14.071865952161918, -11.308101384151682, -9.680739015687942, -9.751119427338061, -10.65282205742676, -11.577126385613825, -11.757477028287855, -11.912305020940494, -12.193423517287698, -11.918699881826493, -11.95650608067958, -12.767142162504575, -13.909339415348747, -14.716001285325426, -14.607641607535122, -13.748436468890192, -12.779227842323113, -12.151850898897981, -11.590530567532223, -11.075176185829488, -11.069295411076588, -12.114215413809315, -13.394228917180104, -13.471681970425102, -14.28960711678617, -17.768606697956606, -20.873628316228434, -20.591151713491897, -18.21588120998991, -15.582458205974813, -13.598506803166394, -13.38687573404677, -14.532082693435306, -14.998920348371339, -14.471537019639582, -13.623440551410654, -13.194904121816828, -13.952254580531806, -14.418612625434617, -13.72716939743817, -13.505604226335066, -13.917715947469471, -13.013278640201854, -11.63267210390307, -12.194600048040904, -13.868010483822658, -15.551300877056317, -16.775780946686954, -15.904668935759936, -14.089430194790094, -14.132843461549953, -15.364639899925951, -15.632837974055114, -14.694050146984445, -13.621922064514168, -13.509825727944278, -13.956778461663689, -13.927379621008377, -14.23883324834247, -15.030429522467443, -15.184780406528018, -14.480651953261287, -13.37481869464809, -13.152725021994561, -14.092992769045587, -14.370099416126408, -13.634517975561634, -12.848636260216932, -13.036311197462242, -14.256261980459573, -14.855728931850381, -15.209523678627798, -16.22194190406387, -16.86326523273269, -16.154127194388963, -14.588353486654398, -13.348507224045356, -12.994386745544126, -13.269062990015785, -13.157915031622792, -12.180516399836732, -10.026861503831599, -7.052971791167542, -5.845726303175387, -7.065655933704698, -8.911125000939101, -11.513610661502906, -16.085771359384218, -20.407630241165297, -21.396167138384726, -20.106500452257777, -17.975292303250065, -14.052713135740255, -9.893299871372655, -8.646128848349901, -9.149649038380884, -9.942465027564314, -11.303147630636158, -12.712263786892503, -13.29433715314628, -13.080522581482215, -13.465960398179956, -14.193519399431707, -13.677047529547702, -12.459438149125262, -12.06940874373609, -12.107555287326452, -11.785374630635854, -11.761797498768441, -11.651700172023837, -10.77470987736827, -10.277467825915608, -10.979673278610102, -12.881408081258911, -15.123729874220714, -16.213375242127398, -15.516951420075724, -13.911355183609802, -13.215512246383728, -13.485188270885878, -13.09270925438608, -12.242260189080177, -12.15706189736493, -12.653112418190535, -13.637348129567245, -14.399944283692626, -13.52164431422721, -11.75595893318745, -11.06743895840709, -11.787906478056772, -13.282462865635717, -15.037174738743053, -15.998085349678094, -15.538088020614815, -14.295939478002916, -13.180531971123715, -12.738227348669096, -13.181176418467498, -13.648596607647516, -13.258217387726916, -12.539095453937708, -12.088858272339287, -12.685126481437479, -14.276052257156362, -14.893817882725962, -14.36015787055838, -14.041620802517395, -14.407343210100926, -15.444115062987073, -16.00679225193796, -15.508281264979395, -14.75309046322542, -13.81673578444708, -13.283293467356337, -13.483001745651414, -13.360947257114628, -13.179303755658113, -13.634519887279453, -13.831356387051446, -13.474672616458133, -13.170406838904325, -12.807174757104738, -12.85903141085613, -13.028999693478996, -12.879068557054092, -12.778687104748215, -11.66008180706607, -10.346017883738256, -10.749178916360336, -11.76256623678157, -11.80256137072276, -11.307211225272418, -11.607907501581659, -12.154154457744, -11.787880351344914, -11.06520934753805, -10.994115324548536, -12.046657227914226, -13.941380915154921, -15.669789456476709, -16.374880875555537, -16.463511260164392, -16.312042315106236, -16.13969256265023, -16.613475743699894, -17.410505946841823, -17.41823906413456, -16.08591138034113, -14.339047723257266, -13.624353465567717, -13.435190070208034, -12.714027946453875, -12.097164240851823, -12.732277665749287, -14.903524601502898, -16.73889136907293, -16.67160097125667, -15.801107907384864, -14.807567162861844, -13.770488028618026, -12.44048318162648, -10.458293828966823, -9.716220244713512, -11.434675657060875, -14.278519548173552, -15.996378519028774, -15.886994941707165, -15.50414067786948, -15.472536627569049, -15.570358131141086, -15.77075088554125, -15.829444745462096, -15.622722116605129, -15.603519678921186, -15.947216208818126, -15.9847639985132, -15.124550300660953, -14.496279264610392, -15.655143644609138, -17.25004835753632, -17.391140085301487, -16.1138480811815, -13.788633252718995, -11.436377252570274, -10.28661385581536, -10.865371519497984, -13.64927432910638, -16.373937066476795, -16.159815741510023, -14.073408578500842, -12.958747399285668, -13.579614544935648, -14.634158502818572, -15.616698511715299, -15.508113952626893, -13.613760018175968, -12.449727291475458, -13.741077336409152, -15.444215816458026, -15.740820503096185, -15.843273548502562, -16.42678541479684, -15.771201787820232, -14.763345515486463, -15.105599187289858, -15.178444696731772, -14.840146325591009, -15.277962309548917, -15.901136374424986, -16.440362928888103, -16.936288057480688, -16.93121534903103, -15.784813648063682, -13.631724859607168, -11.886276109906028, -11.153609655764162, -11.43518563998699, -12.237773393998713, -13.095863869612034, -13.930243295991936, -14.13798038594174, -13.66518602540712, -12.857292312022686, -11.86267664283347, -11.487135120297612, -12.44092046313589, -13.758231634417674, -13.901227486163899, -13.108786179649282, -13.192679723469151, -14.121708854911326, -14.676748186508062, -15.085630055499376, -18.21504665612564, -23.469971789188087, -23.96413629777715, -19.261309800659447, -14.760352028259971, -12.572572541724341, -11.717340299483824, -11.737910510629993, -13.311585653957652, -14.788404070551195, -14.875154861878734, -14.952826851464643, -15.87581943152175, -16.42724129930399, -15.956045118058066, -15.523251954635352, -15.272276040774159, -15.375180213649712, -16.532168565585213, -17.295793035023163, -16.849033721701527, -15.978021366002611, -14.329432083449014, -12.772571435088384, -12.63532748368441, -13.415410486603104, -14.587152070491934, -15.431852962540443, -14.763722270717276, -13.559342430678292, -13.427601042100644, -13.997747235292175, -14.188675725698022, -13.397587518181886, -12.295206354497989, -11.714829641154736, -11.339843470310033, -10.593975584790256, -10.699177499342806, -12.609082611086368, -14.960477551778053, -16.247865706131183, -16.287304292765796, -15.700095818172116, -14.05938236117072, -12.02482152689761, -11.922727610554938, -12.992814852583335, -12.961792282780886, -12.185323884383957, -11.756496533286857, -11.51338595592265, -11.720014774658594, -12.874542808776022, -14.089428151065551, -14.557097139409045, -14.690688982261467, -15.051275208554447, -14.760922111062376, -12.804882009726088, -10.959863009382014, -11.336841875146279, -12.795422656411292, -13.849664037068719, -14.845574113696582, -15.33548227205372, -14.489091358376854, -13.430172559859205, -13.885517522128316, -14.86305594830933, -14.461333485663175, -13.659108700675612, -13.91535106399719, -14.033822650884375, -13.083793883686823, -12.636763007936601, -13.117760949772366, -13.817891523172047, -14.415279383720529, -13.96407661867457, -12.558500701850381, -11.578974086396155, -11.80741035304842, -12.739815294242774, -13.54274968099918, -13.305544323000762, -11.935580514742318, -10.723034702342199, -10.134121222769533, -10.666487717550297, -12.536285030709651, -14.121691345221883, -14.407374544445288, -13.855357257383675, -13.044420489082281, -12.366236661192442, -12.09478214544145, -12.650700087203319, -13.948726898222487, -14.791950185404366, -14.177962391580756, -12.829859354393124, -11.861149292827399, -11.5924705130499, -12.638371813427852, -14.10454090103706, -14.55243816890359, -14.388365660607171, -13.986746454083598, -13.955680289812419, -14.743681408656194, -15.985126741058364, -16.99053665840021, -16.841213597600923, -15.68187631608398, -14.540985925488581, -15.218624931416239, -17.409378785252464, -17.979757709695825, -16.029905519296086, -13.806178790415201, -13.335890583930016, -13.926634072480121, -14.152199745546865, -14.167950605401366, -13.91234995492033, -13.47085491811875, -13.725596060062536, -13.722409032465995, -14.122645924740036, -16.35604561390142, -17.54725415338212, -16.46140367769323, -14.259535934744788, -11.666865620447712, -10.63984603116789, -11.316834698114544, -12.395076670391527, -14.06466971832568, -15.66988744067283, -15.650459477653264, -14.023128242027186, -12.202448408289744, -11.02833874442465, -10.430639742498427, -10.746648971981926, -12.024866914906966, -13.515170230532556, -13.224965075370783, -10.990123165228077, -10.639557297502495, -12.811347244002373, -13.999475001843168, -13.321780810007471, -12.579695231383651, -12.88699688567723, -13.424085523379613, -13.242237224744981, -12.891759458695137, -13.11009731622383, -13.823298436189425, -14.42293161471654, -15.629217146849658, -17.152422764725593, -15.648011719686652, -11.281127354763935, -8.446508223820306, -8.69409789343333, -10.653449299697224, -12.711106850101796, -13.705074638868076, -13.9563106070234, -14.350010917804523, -14.539818734826374, -14.197013532199218, -14.201068707071617, -14.807315728171318, -15.572801322014476, -15.7995325019106, -16.051028062524303, -16.60308758277455, -15.965800634104038, -13.03305729209984, -8.918372168503772, -7.5786881117206715, -10.030329328495204, -13.666999843086876, -16.76662731126304, -17.890974171304848, -16.550974379638504, -14.327041736029882, -12.774595601926109, -13.028556960705, -14.761786800053638, -17.385179579787724, -20.061843315861786, -19.270185004150434, -15.386066467097555, -12.280863714504841, -11.33137417299727, -11.959409797262982, -12.379868611403102, -11.785887191396167, -11.378616418848623, -12.071311315228021, -12.860147250774784, -13.4706016772778, -14.759509047587892, -15.771217761243667, -15.319119364444152, -13.774592086869017, -12.46909727020089, -12.53415596266858, -13.323552043863451, -14.046115575780863, -14.366591906787292, -13.939730013944978, -13.33282424525978, -12.805284223831354, -12.217323425913849, -11.838835343350897, -12.166135654307745, -13.381928624480668, -14.90724449048842, -16.135323902713765, -16.784729654338022, -16.597111172798378, -16.39901633403579, -16.860576660433132, -17.166509376441343, -16.910567773325923, -15.88386863322424, -14.317783758092258, -13.476391043446926, -13.790933113895594, -14.270319387149836, -14.617441743168042, -14.784916414539193, -13.557901648746201, -11.857080778255735, -11.345953915941568, -11.821523470671059, -12.440270367542567, -12.47458305970277, -12.691208702239866, -13.372163117298053, -13.649071330394316, -13.487895946494772, -13.243635599575072, -13.067069863965717, -12.493866842950446, -12.207563243153844, -13.007380950740231, -13.563997631522197, -14.40796140595694, -16.189692064921566, -16.709522925272108, -15.33650999265748, -13.57585081331567, -12.66644961623942, -13.274623994764674, -14.151150030055584, -13.505617960276554, -12.702460216098547, -13.722510356668963, -15.440097464814226, -16.524175260679264, -16.973724572350754, -15.86463158748947, -14.278594631098585, -14.617428404017648, -14.87977649655583, -13.452078892264534, -12.994894047492432, -14.016065972975605, -13.76439602445883, -12.308049023234638, -12.385716906767918, -13.920702619389875, -14.56096314993551, -13.67663393351657, -12.434198029817429, -11.850487850510133, -12.202461281717861, -13.02176829363972, -13.579262802304171, -14.124664547211532, -14.453042740716675, -13.897422578411199, -13.361750540807073, -13.432445112950978, -13.580022867689252, -13.597964578873759, -13.565687601487207, -13.431644932039573, -13.608920502602185, -14.60178698669865, -15.57640970107221, -16.066706240678208, -15.71593264846154, -14.440739370800237, -14.136448733097923, -15.15330485093087, -16.31106727831706, -16.28261554008057, -15.381714810204667, -15.32286995275782, -15.27479751358484, -14.956196116950478, -17.307878955255, -21.779150868318638, -22.770035352446694, -20.456466919344066, -18.725967437755926, -16.889315628384253, -14.855857200359601, -14.331960062029815, -14.906368870913008, -15.720190141873546, -16.881785029032788, -17.705673434315173, -17.314195992847743, -15.791798396589016, -14.096436366691364, -13.786548165071054, -14.254765589212006, -14.506608058511675, -14.783237086783744, -14.471942581347065, -14.086241630935856, -15.388461289692016, -17.818714543879626, -18.50433319042274, -16.192772626766324, -13.101455367774097, -11.93376442286119, -12.449080366181448, -13.714679503537416, -14.44323261333488, -13.439048745214372, -12.73759944302944, -13.289674311198585, -14.14162299553814, -14.956085107916671, -15.92813982140241, -17.354163006898926, -18.374612321862113, -18.470835808902187, -17.537988900277007, -15.454845029479472, -13.606524976841394, -13.534604139120798, -14.082903207252361, -13.549876336435354, -12.86456742717903, -12.68902083367455, -12.361425929433766, -12.111082022907503, -12.374778117494433, -12.316316856791687, -11.0017274781694, -9.781807812937476, -10.14379478440981, -12.160923210651106, -14.52781424274639, -15.891702220289256, -16.974410897483555, -18.02872446658316, -18.173682575105737, -17.275495023540202, -15.989832017628958, -15.07709316175011, -15.328526561692739, -16.45561296743422, -17.239166942221672, -17.114057880949268, -15.856239612094956, -14.712060195976148, -14.93126990999238, -15.90986024082704, -17.149938439821934, -17.70000538234478, -16.438419048436312, -13.796424450391797, -11.335532541762676, -10.872356995344017, -12.134647861657522, -12.990983587641482, -13.084687811810946, -13.668636343100237, -15.164264286206702, -16.770230615131766, -17.492914324003063, -16.46737207403548, -14.28327626923969, -12.858831632266082, -12.927301794790935, -13.6619331079648, -14.526988910621771, -15.097694238448508, -14.956884155632348, -14.92678524594523, -15.140606561898139, -15.44986327469504, -15.865421673581238, -15.665972953735125, -14.851256066347752, -14.149616525204713, -14.052569936492812, -13.804429090496946, -12.528886717894194, -11.018483159663967, -10.800690402896915, -12.368025223560894, -15.187524197449937, -18.006745893107272, -18.553327731447165, -16.566812298374366, -13.633033984277372, -11.529213074773608, -11.792841752314688, -13.816608691937986, -16.222544672449573, -18.011556034344707, -18.89627346166195, -18.938793784874516, -17.902927937442033, -15.838189007229772, -14.139192018192187, -14.397181480631414, -15.499641826944663, -15.37911311963875, -14.019311126075765, -12.972715893427539, -13.122661286962494, -14.491575893720597, -16.513267747783445, -18.45118760285642, -19.506747606455196, -18.684392961502375, -16.873798721756202, -15.733765535684835, -15.457725499277505, -15.772745665013455, -15.868869652205646, -14.68291661927757, -13.239854829063788, -12.469902949206967, -11.834481660281504, -11.98020671517688, -13.403346513141763, -14.8917827096755, -15.332558516241477, -14.763825168448841, -14.568848321734468, -15.648541972666536, -16.340954899390894, -15.755190527130534, -15.069753344756524, -14.325878543717774, -13.36487035159563, -13.194936770730447, -13.843213282952139, -14.803951985888549, -15.493652950874255, -14.456828001209068, -12.468351158962422, -11.622623040235517, -11.976243901950907, -13.27496773114191, -14.967329116876371, -15.934732644031868, -15.696902536754061, -14.954944172991311, -14.529957967459929, -13.497916928484512, -12.178406009476117, -11.571266083040669, -10.95053067920557, -10.9581999952695, -12.051022153516044, -12.785895107650685, -13.212096993411912, -13.954752771095617, -14.122343766073959, -14.618584583159612, -16.299785195508885, -16.743111998471683, -15.136218218496996, -13.766341851700732, -13.791489870729734, -14.271825106046906, -14.423413617071265, -14.210958744883634, -14.350649158533457, -15.236586344838784, -15.341874952579886, -14.07188780618268, -13.034698385161661, -13.456466599367024, -14.687998656867855, -15.122722373315773, -15.610228502628503, -17.487042950693663, -19.19164961153492, -18.513435127752444, -15.450815774211463, -12.496528832549519, -11.31785994799672, -11.679517945185294, -12.511013076017232, -12.10045973535152, -10.752803779544799, -10.400121256526083, -11.200245147516357, -12.3650632461475, -14.270498119987941, -16.557366304087125, -17.78540812820193, -17.98566552284293, -16.788812001071022, -14.519713412098806, -12.974600065974304, -12.860005866929985, -13.462265347875285, -12.79907515004551, -11.484904910238816, -11.833791746377033, -13.18656859420624, -14.248052152598609, -15.481320343563288, -15.899704600151617, -14.51623664200101, -13.560584488143856, -13.999422639370518, -15.122238225841825, -16.717977039618745, -17.75055108615614, -17.313478638968576, -15.580900705709768, -14.38599459953044, -14.12984551534934, -13.603230367618822, -13.973164456467321, -14.399848969862132, -13.800139967603945, -14.9474911126437, -17.010175730311985, -16.229297305594343, -13.731574724855435, -12.515671757050683, -12.787668076524437, -13.547040728007405, -13.97705654405547, -13.738830834536618, -12.980366584564315, -11.8565328371242, -11.049793635460041, -10.566172798141265, -10.281492694303203, -11.248242466535075, -12.645120552439975, -13.932753136555123, -15.266905188086497, -15.802651724930369, -16.155934272166046, -15.72464363535812, -13.540529834404465, -11.429828994748199, -11.046558749136995, -12.169823626260003, -13.161342511164573, -12.84305419860394, -12.40772495059932, -12.884437287204866, -13.869520029476426, -15.127516198083747, -15.594681154280531, -14.932378932125989, -14.44512597556665, -14.499400108783213, -14.615356831552447, -14.901852646348287, -15.621466614679235, -16.497319784351905, -17.37610396785408, -17.61978536628823, -17.4589712578921, -17.71428249435997, -17.12991728287773, -15.517558003038795, -14.680354864244402, -14.916640633316899, -15.223218559851452, -15.531132150851361, -16.109767518045164, -16.45504123741018, -16.099534601427834, -15.356375272079461, -15.067113367841321, -15.139745478527633, -15.207013251000108, -14.953329992718686, -13.813052875848445, -12.822550386247865, -12.464050201508607, -12.651482628336757, -14.314530697745202, -16.698669635000055, -17.903952660273212, -17.171649612765183, -14.907893794718317, -12.72481213855229, -12.885634381356567, -14.350739368975526, -15.09265974627466, -15.499042802795573, -15.244353338644933, -13.892458060829536, -12.214620092994211, -11.669157483508098, -11.909431871927053, -11.243843805301754, -10.731492041187616, -11.15372236495011, -12.113113144946158, -13.755571661923096, -14.49614411079798, -13.963458828653424, -13.214380845371547, -12.68570511059819, -13.51089931119878, -15.34380476595091, -16.503926648709317, -16.596207272442506, -16.198871911670366, -15.207713895456155, -13.819899838763327, -13.525259714048108, -14.49112360952055, -15.20706897920126, -15.755376261066536, -16.2289390132898, -15.418707361571295, -13.813541873249306, -12.66788562780117, -12.610961088510791, -13.329701825080576, -14.123943009439866, -14.828442679603025, -16.399477152225145, -18.32924694482739, -18.355769247732397, -16.565945241926922, -14.576748999964439, -13.590818018309758, -13.324338788417343, -12.91358805694342, -12.615154963437497, -12.861230746815387, -13.290341991071575, -13.515255617937061, -13.29137591868867, -12.810066759179819, -13.114328208779462, -14.440304697410177, -15.491395763678753, -15.942750688668177, -16.506083868843696, -16.203330332308486, -14.558540958713163, -12.522950073674224, -11.737826144456161, -13.04296952136936, -14.828071692903542, -16.271296513944982, -16.841685721204808, -16.312592445056147, -15.818890930585274, -15.529789104282264, -14.836002022369286, -13.106687688789417, -11.609905787052705, -11.751475117390399, -10.724147022679501, -7.365237279027941, -6.005335595159389, -7.990728177794618, -10.511136962958226, -12.420865772423898, -13.4788701721745, -14.327945381160166, -14.873424104862648, -14.128370578519931, -14.122780792627612, -15.14691045089794, -14.94275953917785, -14.506538733941966, -14.553840410297337, -14.15805735589889, -13.866773361193097, -13.431182643302364, -12.434180930382965, -11.737026679871146, -11.11918403460425, -10.378536860790977, -10.764875213560279, -11.961787334559093, -12.961467453292842, -14.09079063855215, -14.919931115176116, -14.83705582683666, -13.896753659164942, -13.330746588591435, -14.282116935999744, -15.660639743767318, -16.838462207697212, -17.098891981728315, -15.292091799462487, -13.01365896192402, -13.51805114117139, -16.119909281911355, -16.54984354968057, -14.232913031887493, -11.61228534959158, -10.401999413389527, -10.622628815293012, -11.917486366211866, -13.55290200350023, -13.58922566712478, -13.273595545726238, -14.135481600855007, -14.467499169283183, -14.005077618362682, -14.044216313949946, -14.723412511687934, -14.86256323137196, -13.98630847195084, -13.406677207624737, -14.226222332957477, -15.582631600298992, -15.51434301087404, -13.826250613626321, -12.452726847492524, -12.501502271205508, -13.102960510004857, -13.263238009356645, -12.823338713556616, -12.062278628160055, -11.296115251185332, -11.120349405990156, -12.381596445517552, -14.31271768368237, -15.029563057008122, -14.768811058194185, -14.479285404202193, -13.902711041035293, -13.357988996689965, -12.74371836370764, -12.34615247173534, -13.445284580011625, -14.711709306516244, -15.24643540090901, -15.914224859597738, -15.38927003828023, -13.20727530602315, -11.910842321832813, -12.58745803520579, -12.974104264949052, -12.332050671617749, -12.574145391441832, -13.40693663840629, -13.33035293235088, -12.882920966584676, -12.584237038723748, -12.158885900736502, -12.052684457157518, -12.387233707398053, -13.030943465385779, -13.819215647437812, -14.347835868574851, -14.778728544484252, -15.008771314904115, -13.910453951582934, -11.724327685127873, -10.712751373412452, -11.561678638277932, -12.601615970205959, -12.90857824272, -13.827650000739647, -15.17762484418552, -15.36298749631886, -15.08775746623985, -14.668849481717523, -13.6822250791139, -12.989293739472298, -12.567235535192681, -11.521612700897478, -9.797796450292143, -8.911632139711678, -9.43180241574007, -10.022349612793057, -10.600994903521732, -11.340222141556549, -12.137183720596738, -12.349264004950955, -11.502512771398802, -10.82875677019263, -10.866308223370595, -11.126297406686719, -11.847055773060461, -13.416240945946345, -15.338847636633144, -15.847388300220992, -14.709665409589984, -13.858020718710177, -13.239061221601364, -11.8654403726647, -10.2885426842621, -9.943120412863218, -9.94782358914977, -9.09108781403167, -8.67230614532593, -9.832257541518993, -13.213347699846118, -16.795468189625915, -17.28833440977025, -15.485031172836777, -13.91346505510704, -13.130510461783064, -13.01382023756341, -14.043468159986563, -15.346019491113307, -15.547443178518575, -14.912639183399545, -13.661212570406912, -12.204802211818294, -11.736982926507139, -12.562437377521402, -13.887147350873462, -14.763313334614484, -14.757276263143535, -13.971373764973286, -12.353750484613068, -11.18823920234372, -11.995427408603792, -13.73074194610755, -14.707225154883597, -14.951793100964982, -15.345034933575402, -16.22005067782192, -17.40209818684314, -17.93197813236561, -16.47544073261172, -13.85163565189784, -12.156294183849923, -11.725405831590082, -11.981905292787566, -12.172102608843126, -12.07066039183015, -12.790300303520695, -13.893121683034785]
  in  "stop":bool
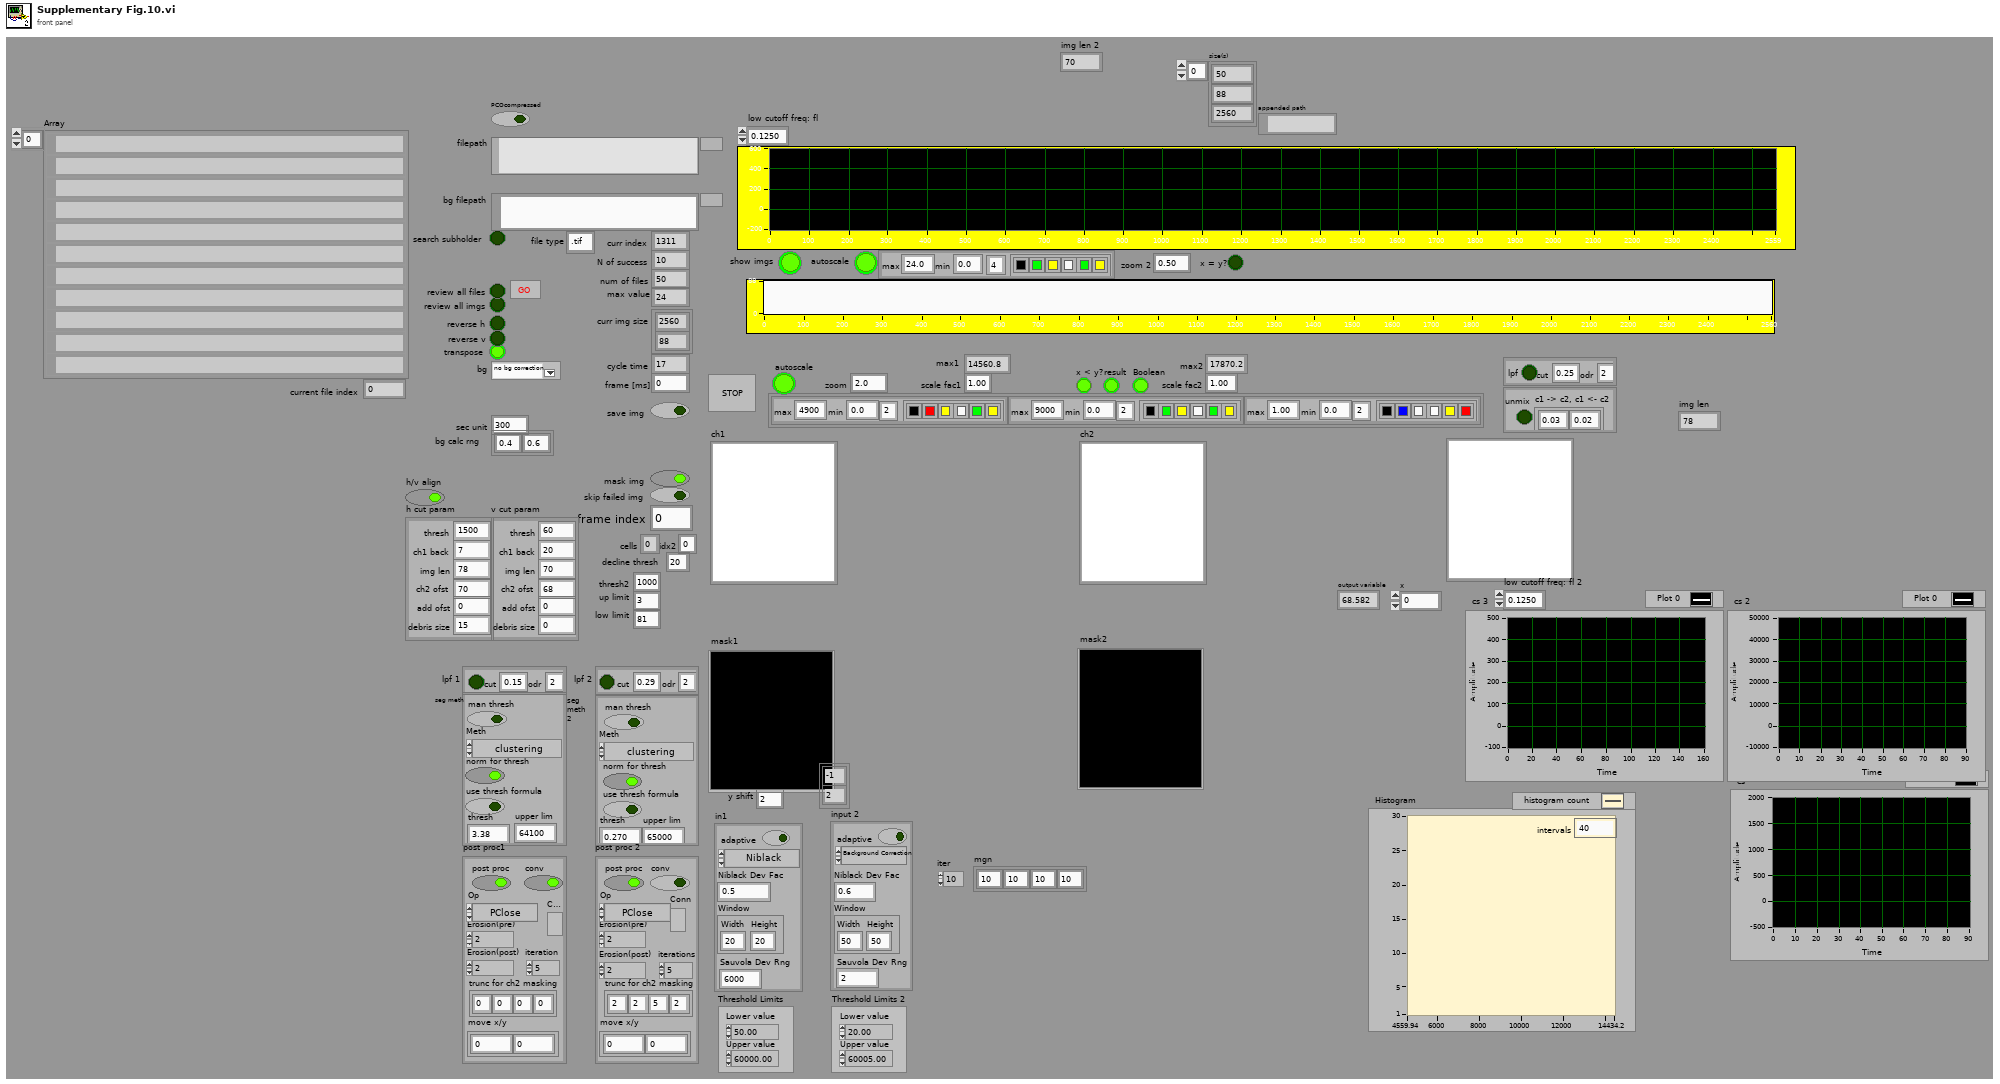
[diagram p1: front panel]
types:
  T1 = cluster{"thresh":dbl, "ch1 back":dbl, "img len":i32, "ch2 ofst":i16, "add ofst":i32, "debris size":dbl}
  T2 = cluster{"X Values":dbl[], "Histogram: h(x)":i32[]}
  T3 = cluster{"color array":u32[], "num of colors":i32, "max":dbl, "min":dbl}
  T4 = cluster{"Niblack Dev Fac":dbl, "Window":cluster{"Width":i32, "Height":i32}, "Sauvola Dev Rng":dbl, "adaptive":bool, "Method (Niblack)":u32}
  T5 = cluster{"trunc for ch2 masking":i32[], "Erosion(pre)":i32, "Op":enum32{"AutoM", "Close", "Dilate", "Erode", "Gradient", "Gradient out", "Gradient in", "Hit miss", "Open", "PClose", "POpen", "Thick", "Thin"}, "post proc":bool, "move x/y":i32[], "conv":bool, "Conn":bool, "iterations":i32, "Erosion(post)":i32}
  T6 = cluster{"trunc for ch2 masking":i32[], "Erosion(pre)":i32, "Op":enum32{"AutoM", "Close", "Dilate", "Erode", "Gradient", "Gradient out", "Gradient in", "Hit miss", "Open", "PClose", "POpen", "Thick", "Thin"}, "post proc":bool, "move x/y":i32[], "conv":bool, "Conn":bool, "iteration":i32, "Erosion(post)":i32}
  T7 = cluster{"norm for thresh":bool, "use thresh formula":bool, "thresh":dbl, "man thresh":bool, "Meth":i32, "upper lim":i32}
  T8 = cluster{"color array":u32[], "num of colors":i32, "max":dbl, "min":dbl}[]
  T9 = cluster{"c1 -> c2, c1 <- c2":dbl[], "unmix":bool}
  T10 = typedef "LVBoundsTypeDef.ctl" = cluster{"Width":u32, "Height":u32}
  T11 = cluster{"color array":u32[], "num of colors":i32, dbl, "min":dbl}
  T12 = enum16{"open", "replace", "create", "open or create", "replace or create", "replace or create with confirmation"}
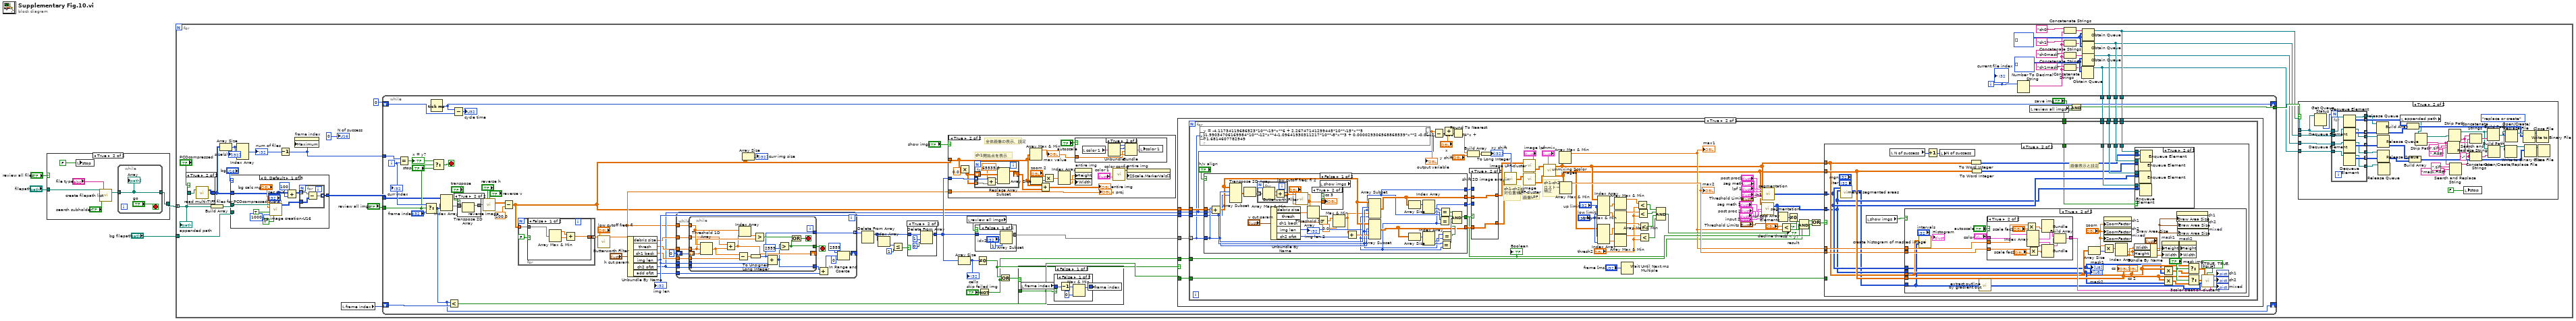
[diagram p0: block diagram]
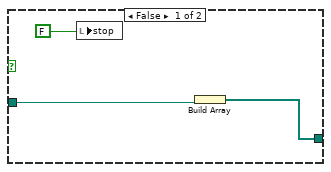
[diagram p2: hidden frame]
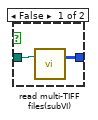
[diagram p3: hidden frame]
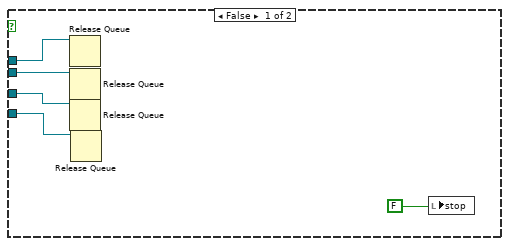
[diagram p4: hidden frame]
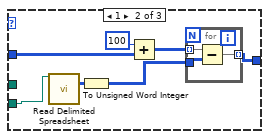
[diagram p5: hidden frame]
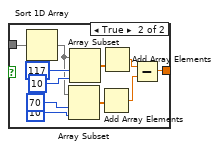
[diagram p7: hidden frame]
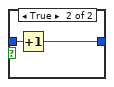
[diagram p11: hidden frame]
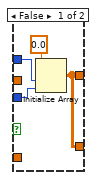
[diagram p15: hidden frame]
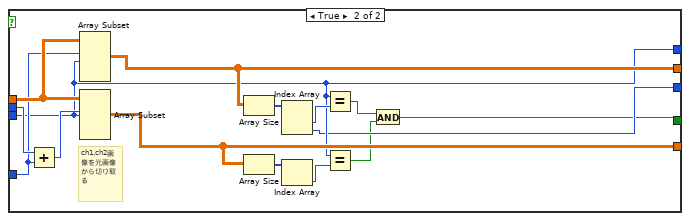
[diagram p17: hidden frame]
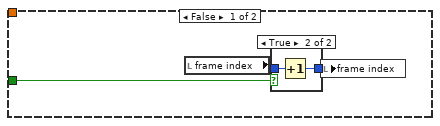
[diagram p18: hidden frame]
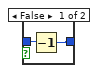
[diagram p19: hidden frame]
diagram:
  n1 = case shown="True" "review all files" {
    tunnel: "filepath" -> [w7 w11]
    tunnel: [w6 w10] -> w3
    frame False {
      n2 = local write "stop"(FALSE) -> ()
      n3 = Build Array(w7) -> (w6:path[])
    }
    frame True {
      n4 = local write "stop"(FALSE) -> ()
      n5 = call "create filepath list.vi"("regular expression"="file type", "search subholder"="search subholder", "path"=w11) -> ("Array"=w9:path[])  [unwired: 1 out]
      n6 = while {
        tunnel: [w15] -> w10
        tunnel: w9 -> [w15]
        stop <- "go" stop-if-true
        "Array" <- w15
      }
    }
  }
  n7 = for {
    tunnel: w3 -> [w25] mode=indexing
    tunnel: "bg filepath" -> [w23]
    i -> [w22]
    w34 = u8[][] [] ("Array")
    w35 = i16[][] [] ("16bit integer")
    n8 = case shown="True" "PCOcompressed" {
      tunnel: [w48 w49] -> w40
      tunnel: w25 -> [w47 w50]
      frame False {
        n9 = call "read multi-TIFF files(subVI).vi"("file path (use dialog)"=w47) -> ("image data"=w48:u16[][][])  [unwired: 2 in]
      }
      frame True {
        n10 = call "read multi-TIFF files for PCOcompressed(subVI).vi"("file path (use dialog)"=w50) -> ("Array"=w49:i32[][][])  [unwired: 2 in]
      }
    }
    n11 = Build Array(w25) -> (w39:path[])
    n12 = Array Size(array=w40) -> (size(s)=w43:i32[])
    "size(s)" <- w43
    n13 = case shown="0, Default" "bg" {
      tunnel: w39 -> [w115 _ _]
      tunnel: [w114 w123 w129] -> w38
      tunnel: w40 -> [w108 w124 w129]
      tunnel: w23 -> [_ w122 _]
      frame 0, Default {
        n14 = call "bg image creation-U16.vi"("Array in"=w115, "section unit"="sec unit", "input array"=w108, "Array"="bg calc rng", "partial select"=TRUE, "length"=1000, "save"=TRUE) -> ("created bg image"=w107:u16[][])  [unwired: 6 in, 2 out]
        n15 = Add(x=w108, y=u16 100) -> (x+y=w106:i32[][][])
        n16 = for {
          tunnel: [w118] -> w114 mode=indexing
          tunnel: w106 -> [w117] mode=indexing
          tunnel: w107 -> [w116]
          n17 = Subtract(x=w117, y=w116) -> (x-y=w118:i32[][])
        }
      }
      frame 1 {
        n18 = call-poly <vilib>:"Read Delimited Spreadsheet.vi"("file path (dialog if empty)"=w122) -> ("all rows"=w125:i64[][])  [unwired: 9 in, 5 out]
        n19 = To Unsigned Word Integer(number=w125) -> (unsigned 16bit integer=w121:u16[][])
        n20 = Add(x=u16 100, y=w124) -> (x+y=w120:i32[][][])
        n21 = for {
          tunnel: [w128] -> w123 mode=indexing
          tunnel: w121 -> [w127]
          tunnel: w120 -> [w126] mode=indexing
          n22 = Subtract(x=w126, y=w127) -> (x-y=w128:i32[][])
        }
      }
      frame 2 {
      }
    }
    n23 = Index Array(array=w43) -> (element #1=w42:i32)  [unwired: 3 in, 2 out]
    "num of files" <- w42
    n24 = Decrement(x=w42) -> (x-1=w44:i32)
    n25 = property on="frame index" class="DigNum (strict)"("Maximum"=w44) -> ()  [unwired: 2 in, 2 out]
    n26 = local read "frame index"() -> (w24:i32)
    n27 = Number To Decimal String(number=w22) -> (decimal integer string=w17:string)  [unwired: 1 in]
    n28 = Concatenate Strings("ch0" ("name (unnamed)"), w17) -> (w21:string)
    n29 = Concatenate Strings("ch1" ("name (unnamed)"), w17) -> (w20:string)
    n30 = Concatenate Strings("ch0mask" ("name (unnamed)"), w17) -> (w19:string)
    n31 = Concatenate Strings("ch1mask" ("name (unnamed)"), w17) -> (w18:string)
    n32 = Obtain Queue(name (unnamed)=w18, element data type=w34) -> (queue out=w26:refnum<queue>)  [unwired: 3 in, 2 out]
    n33 = Obtain Queue(name (unnamed)=w21, element data type=w35) -> (queue out=w29:refnum<queue>)  [unwired: 3 in, 2 out]
    n34 = Obtain Queue(name (unnamed)=w20, element data type=w35) -> (queue out=w28:refnum<queue>)  [unwired: 3 in, 2 out]
    n35 = Obtain Queue(name (unnamed)=w19, element data type=w34) -> (queue out=w27:refnum<queue>)  [unwired: 3 in, 2 out]
    n36 = while {
      shift-right: [w184] -> _
      shift-left: 0 -> [w183]
      tunnel: "review all imgs" -> [w175]
      tunnel: w44 -> [w180]
      tunnel: w38 -> [w143]
      tunnel: [w136] -> w37
      tunnel: w29 -> [w140]
      tunnel: w28 -> [w139]
      tunnel: w27 -> [w138]
      tunnel: w26 -> [w137]
      shift-right: [w134] -> _
      shift-left: w24 -> [w135]
      i -> [w177]
      stop <- w179 stop-if-true
      n37 = Equal?(x=w180, y=w177) -> (x = y?=w176:bool)
      "x = y?" <- w176
      n38 = Select(t=w177, s=w175, f="frame index") -> (s? t:f=w134:i32)
      n39 = Tick Count (ms)() -> (millisecond timer value=w184:u32)
      n40 = Select(t=w176, s=w175, f="stop") -> (s? t:f=w179:bool)
      n41 = Index Array(array=w143, index (dim 0)=w134) -> (element=w174:i32[][])  [unwired: 2 in]
      n42 = Less?(x=w134, y=w135) -> (x < y?=w172:bool)
      n43 = Subtract(x=w184, y=w183) -> (x-y=→"cycle time":u32)
      n44 = case shown="True" "transpose" {
        tunnel: [w500 w502] -> w142
        tunnel: w174 -> [w500 w501]
        frame False {
        }
        frame True {
          n45 = Transpose 2D Array(2D array=w501) -> (transposed array=w502:i32[][])
        }
      }
      n46 = call "reverse image.vi"("output array in"=w142, "reverse h"="reverse h", "reverse v"="reverse v") -> ("output array out"=w130:dbl[][])
      n47 = Subtract(x=w130, y=100.0) -> (x-y=w132:dbl[][])
      n48 = for {
        tunnel: w132 -> [w187] mode=indexing
        tunnel: [w186] -> w154 mode=indexing
        n49 = case shown="False" FALSE {
          tunnel: w187 -> [w191 w202]
          tunnel: [w188 w194] -> w186
          frame False {
            n50 = Array Max & Min(array=w191) -> (max value=w189:dbl, min value=w190:dbl)  [unwired: 2 out]
            n51 = Add(x=w189, y=w190) -> (x+y=w188:dbl)
          }
          frame True {
            n52 = Sort 1D Array(array=w202) -> (sorted array=w195:dbl[])
            n53 = Array Subset(array=w195, index=70, length=10) -> (w198:dbl[])
            n54 = Array Subset(array=w195, index=117, length=10) -> (w199:dbl[])
            n55 = Add Array Elements(numeric array=w198) -> (sum=w192:dbl)
            n56 = Add Array Elements(numeric array=w199) -> (sum=w193:dbl)
            n57 = Subtract(x=w193, y=w192) -> (x-y=w194:dbl)
          }
        }
      }
      n58 = call-poly <vilib>:"Butterworth Filter.vi"("low cutoff freq: fl"="low cutoff freq: fl", "X"=w154) -> ("Filtered X"=w145:dbl[])  [unwired: 6 in, 1 out]
      n59 = Unbundle By Name("h cut param") -> ("debris size"=w149:dbl, "thresh"=w150:dbl, "ch1 back"=w151:dbl, "img len"=w152:i32, "ch2 ofst"=w148:i16, "add ofst"=w147:i32)
      "img len" <- w152
      n60 = while {
        tunnel: w151 -> [w254]
        tunnel: [w253] -> w165 mode=indexing
        tunnel: w148 -> [w255]
        tunnel: w145 -> [w258]
        tunnel: w152 -> [w256]
        tunnel: w150 -> [w257]
        shift-right: [w260] -> _
        shift-left: u32 0 -> [w264]
        tunnel: w147 -> [w263]
        tunnel: w149 -> [w250]
        stop <- w251 stop-if-true
        n61 = while {
          tunnel: w258 -> [w280]
          tunnel: w256 -> [w266]
          tunnel: w255 -> [w273]
          tunnel: w254 -> [w274]
          tunnel: [w270] -> w253
          tunnel: [w265] -> w252
          tunnel: [w269] -> w251
          tunnel: w257 -> [w278]
          shift-right: [w268] -> _
          shift-left: w264 -> [w281]
          tunnel: w250 -> [w267]
          stop <- w271 stop-if-true
          n62 = Threshold 1D Array(1:w281, 2:w278, 3:w280) -> (0:w276:dbl)
          n63 = Add(x=w267, y=w276) -> (x+y=w268:dbl)
          n64 = Subtract(x=w276, y=w274) -> (x-y=w275:dbl)
          n65 = Index Array(array=w280, index=w268) -> (element=w279:dbl)
          n66 = To Unsigned Long Integer(number=w275) -> (unsigned 32bit integer=w270:u32)
          n67 = Greater?(x=w279, y=w278) -> (0:w277:bool)
          n68 = Compound Arithmetic op=ADD(w270, w273, w266) -> (w265:u32)
          n69 = Greater?(x=w265, y=u32 2559) -> (0:w269:bool)
          n70 = Or(x=w277, y=w269) -> (x .or. y?=w271:bool)
        }
        n71 = Add(x=w252, y=w263) -> (x+y=w262:u32)
        n72 = In Range and Coerce(upper limit=u32 2559 ("y"), x=w262, lower limit=u32 0) -> (coerced(x)=w260:u32)  [unwired: 1 out]
      }
      n73 = Array Size(array=w132) -> (size(s)=→"curr img size":i32[])
      n74 = Delete From Array(array=w165) -> (array with subset deleted=w160:u32[])  [unwired: 2 in, 1 out]
      n75 = Index Array(array=w160) -> (element=w162:u32)  [unwired: 1 in]
      n76 = Less Or Equal?(x=w162, y=u32 1) -> (x <= y?=w159:bool)
      n77 = case shown="True" w159 {
        tunnel: w160 -> [w203 w207]
        tunnel: [w203 w204] -> w155
        frame False {
        }
        frame True {
          n78 = Delete From Array(array=w207, length=1, index=0) -> (array with subset deleted=w204:u32[])  [unwired: 1 out]
        }
      }
      n79 = case shown="True" "show imgs" {
        tunnel: w132 -> [_ w212]
        tunnel: w145 -> [_ w214]
        tunnel: w155 -> [_ w211]
        frame False {
        }
        frame True {
          # "ch1開始点を表示"
          # "全体画像の表示、設定"
          n80 = Multiply(x=w212, y=0.0) -> (x*y=w210:dbl[][])
          n81 = for {
            tunnel: w211 -> [w229] mode=indexing
            shift-right: [w227] -> w208
            shift-left: w210 -> [w228]
            tunnel: w210 -> [w225] mode=indexing
            n82 = Add(x=65535.0, y=w225) -> (x+y=w224:dbl[])
            n83 = Replace Array Subset(array=w228, new element=w224, index (row)=w229) -> (w227:dbl[][])  [unwired: 1 in]
          }
          n84 = Array Max & Min(array=w212) -> (max value=w218:dbl)  [unwired: 3 out]
          "max value" <- w218
          n85 = Array Size(array=w212) -> (size(s)=w219:i32[])
          n86 = Add(x=w212, y=w208) -> (x+y=→"entire img":dbl[][])
          n87 = Multiply(x="zoom 2", y=w219) -> (x*y=w221:dbl[])
          n88 = Index Array(array=w221) -> (element #1=w223:dbl, element #2=w222:dbl)  [unwired: 2 in]
          n89 = case shown="True" "autoscale" {
            tunnel: w218 -> [_ w231]
            frame False {
            }
            frame True {
              n90 = local read "color 1"() -> (w234:T3)
              n91 = Unbundle(w234) -> ("color array"=w232:u32[], "num of colors"=w233:i32, "min"=w235:dbl)  [unwired: 1 out]
              n92 = Bundle("color array"=w232, "num of colors"=w233, w231, "min"=w235) -> (w230:T11)  [unwired: 1 in]
              n93 = local write "color 1"(w230) -> ()
            }
          }
          n94 = property on="entire img" class="IntGraph (strict)"("Height"=w222, "Width"=w223) -> ()  [unwired: 2 in, 2 out]
          n95 = call "color config.vi"("color 1"="color 1") -> ("Array"=w217:cluster{dbl, u32}[])  [unwired: 9 in, 1 out]
          n96 = property on="entire img" class="IntGraph (strict)"("ZScale.MarkerVals[]"=w217) -> ()  [unwired: 2 in, 2 out]
          "x proj" <- w214
        }
      }
      n97 = Array Size(array=w155) -> (size(s)=w158:i32)
      "cells" <- w158
      n98 = local read "review all imgs"() -> (w164:bool)
      n99 = case shown="False" w164 {
        tunnel: w155 -> [w248 w249]
        tunnel: [w245 w249] -> w173
        frame False {
          n100 = Array Subset(array=w248, index="idx2", length=1) -> (w245:u32[])
        }
        frame True {
        }
      }
      n101 = Not Equal To 0?(x=w158) -> (x != 0?=w171:bool)
      n102 = Not(x="skip failed img") -> (.not. x?=w170:bool)
      n103 = Or(x=w171, y=w170) -> (x .or. y?=w156:bool)
      n104 = case shown="False" w156 {
        tunnel: w172 -> [w236 _]
        frame False {
          n105 = local read "frame index"() -> (w238:i32)
          n106 = case shown="False" w236 {
            tunnel: w238 -> [w242 w244]
            tunnel: [w241 w243] -> w237
            frame False {
              n107 = Decrement(x=w242) -> (x-1=w240:i32)
              n108 = Max & Min(x=w240, y=0) -> (max(x,y)=w241:i32)  [unwired: 1 out]
            }
            frame True {
              n109 = Increment(x=w244) -> (x+1=w243:i32)
            }
          }
          n110 = local write "frame index"(w237) -> ()
        }
        frame True {
        }
      }
      n111 = local read "review all imgs"() -> (w168:bool)
      n112 = Compound Arithmetic op=AND("save img", w168) -> (w136:bool)
      n113 = case shown="True" w171 {
        tunnel: w152 -> [_ w292]
        tunnel: w148 -> [_ w291]
        tunnel: w173 -> [_ w290]
        tunnel: w132 -> [_ w289]
        tunnel: w172 -> [_ w288]
        tunnel: w170 -> [_ w287]
        tunnel: w140 -> [_ w286]
        tunnel: w139 -> [_ w285]
        tunnel: w138 -> [_ w284]
        tunnel: w137 -> [_ w283]
        tunnel: w136 -> [_ w282]
        frame False {
        }
        frame True {
          n114 = for {
            tunnel: w289 -> [w320]
            tunnel: w292 -> [w319]
            tunnel: w290 -> [w300] mode=indexing
            tunnel: w291 -> [w296]
            tunnel: w288 -> [w348]
            tunnel: w287 -> [w341]
            tunnel: w286 -> [w305]
            tunnel: w285 -> [w304]
            tunnel: w284 -> [w303]
            tunnel: w283 -> [w302]
            tunnel: w282 -> [w301]
            # "ch1-ch2クロストーク補正"
            # "画像LPF"
            # "ch1-ch2相対位置補正"
            n115 = formula code="y = -4.11734119686523*10**-19*x**6 + 2.26747141299445*10**-15*x**5 -1.99034706169984*10**-12*x**4-1.09641930311217*10**-8*x**3 + 0.000029306568868539*x**2 -0.0212100702013434*x + 71.6814607782949\n;"("x"=w300) -> ("y"=w297:dbl)
            "output variable" <- w297
            n116 = case shown="False" "h/v align" {
              tunnel: w296 -> [w402 w420]
              tunnel: [w375 w413] -> w310
              tunnel: [w376 w414] -> w309
              tunnel: w300 -> [w394 w419]
              tunnel: w320 -> [w393 w421]
              tunnel: w319 -> [w373 w412]
              tunnel: [w374 w408] -> w306
              tunnel: [w373 w412] -> w308
              tunnel: [w372 w411] -> w307
              frame False {
                n117 = Add(x=w394, y=w402) -> (x+y=w390:u32)
                n118 = Array Subset(array=w393, index (row)=w394, length (row)=w373) -> (w401:dbl[][])  [unwired: 2 in]
                n119 = Transpose 2D Array(2D array=w401) -> (transposed array=w400:dbl[][])
                n120 = for {
                  tunnel: w400 -> [w407] mode=indexing
                  tunnel: [w406] -> w397 mode=indexing
                  n121 = Array Max & Min(array=w407) -> (max value=w405:dbl, min value=w404:dbl)  [unwired: 2 out]
                  n122 = Add(x=w405, y=w404) -> (x+y=w406:dbl)
                }
                n123 = Unbundle By Name("v cut param") -> ("thresh"=w398:dbl, "ch1 back"=w395:dbl, "img len"=w372:i32, "ch2 ofst"=w392:i16)  [unwired: 1 out]
                "img len 2" <- w372
                n124 = call-poly <vilib>:"Butterworth Filter.vi"("low cutoff freq: fl"="low cutoff freq: fl 2", "X"=w397) -> ("Filtered X"=w388:dbl[])  [unwired: 6 in, 1 out]
                n125 = Threshold 1D Array(2:w398, 3:w388) -> (0:w396:dbl)  [unwired: 1 in]
                n126 = Subtract(x=w396, y=w395) -> (x-y=w370:dbl)
                n127 = local read "show imgs"() -> (w387:bool)
                n128 = case shown="True" w387 {
                  tunnel: w388 -> [_ w403]
                  frame False {
                  }
                  frame True {
                    "cs 3" <- w403
                  }
                }
                n129 = Max & Min(x=w370, y=0.0) -> (max(x,y)=w371:dbl)  [unwired: 1 out]
                n130 = Add(x=w371, y=w392) -> (x+y=w391:dbl)
                n131 = Array Subset(array=w393, index (row)=w394, length (row)=w373, index (col)=w371, length (col)=w372) -> (w376:dbl[][])
                n132 = Array Subset(array=w393, index (row)=w390, length (row)=w373, index (col)=w391, length (col)=w372) -> (w375:dbl[][])
                n133 = Array Size(array=w376) -> (size(s)=w377:i32[])
                n134 = Array Size(array=w375) -> (size(s)=w384:i32[])
                n135 = Index Array(array=w377) -> (element #1=w379:i32, element #2=w378:i32)  [unwired: 2 in]
                n136 = Index Array(array=w384) -> (element #1=w382:i32, element #2=w383:i32)  [unwired: 2 in]
                n137 = Equal?(x=w378, y=w372) -> (x = y?=w381:bool)
                n138 = Equal?(x=w379, y=w373) -> (x = y?=w380:bool)
                n139 = Equal?(x=w383, y=w372) -> (x = y?=w386:bool)
                n140 = Equal?(x=w382, y=w373) -> (x = y?=w385:bool)
                n141 = Compound Arithmetic op=AND(w380, w381, w385, w386) -> (w374:bool)
              }
              frame True {
                # "ch1,ch2画像を元画像から切り取る"
                n142 = Add(x=w420, y=w419) -> (x+y=w422:u32)
                n143 = Array Subset(array=w421, index (row)=w419, length (row)=w412) -> (w414:dbl[][])  [unwired: 2 in]
                n144 = Array Subset(array=w421, index (row)=w422, length (row)=w412) -> (w413:dbl[][])  [unwired: 2 in]
                n145 = Array Size(array=w414) -> (size(s)=w415:i32[])
                n146 = Array Size(array=w413) -> (size(s)=w418:i32[])
                n147 = Index Array(array=w415) -> (element #1=w416:i32, element #2=w411:i32)  [unwired: 2 in]
                n148 = Index Array(array=w418) -> (element=w417:i32)  [unwired: 1 in]
                n149 = Equal?(x=w412, y=w416) -> (x = y?=w410:bool)
                n150 = Equal?(x=w412, y=w417) -> (x = y?=w409:bool)
                n151 = And(x=w410, y=w409) -> (x .and. y?=w408:bool)
              }
            }
            "Boolean" <- w306
            n152 = Subtract(x=w297, y=w296) -> (x-y=w298:dbl)
            n153 = Add(x="x", y=w298) -> (x+y=w295:dbl)
            n154 = Round To Nearest(number=w295) -> (nearest integer value=w299:dbl)
            n155 = Build Array(w299, "y shift") -> (w339:dbl[])
            n156 = case shown="True" w306 {
              tunnel: w309 -> [_ w368]
              tunnel: [w363 w368] -> w312
              tunnel: w308 -> [w366 _]
              tunnel: w307 -> [w365 _]
              tunnel: w310 -> [_ w367]
              tunnel: [w363 w367] -> w311
              frame False {
                n157 = Initialize Array(0.0, w366, w365) -> (w363:dbl[][])
              }
              frame True {
              }
            }
            n158 = To Long Integer(number=w339) -> (32bit integer=w337:i32[])
            "xy shift" <- w337
            n159 = call "shift 2D image arrayin.vi"("Array in"=w311, "shift"=w337) -> ("Array out"=w340:dbl[][])
            n160 = call "image LPF-cluster.vi"("image lpf"="image lpf", "input"=w312) -> ("output"=w361:dbl[][])  [unwired: 1 in]
            n161 = call "image LPF-cluster.vi"("image lpf"="image lpf", "input"=w340) -> ("output"=w360:dbl[][])  [unwired: 1 in]
            n162 = call "unmixing 2color images.vi"("parameters"="unmix", "ch2"=w360, "ch1"=w361) -> ("unmixed ch2"=w313:dbl[][], "unmixed ch1"=w314:dbl[][])  [unwired: 4 in]
            n163 = Array Max & Min(array=w314) -> (max value=w317:dbl)  [unwired: 3 out]
            "max1" <- w317
            n164 = Array Max & Min(array=w313) -> (max value=w344:dbl)  [unwired: 3 out]
            "max2" <- w344
            n165 = Index Array(array=w314, index (col) #1="up limit", index (col) #2="low limit") -> (element #1=w336:dbl[], element #2=w335:dbl[])  [unwired: 2 in]
            n166 = Index Array(array=w313, index (col) #1="up limit", index (col) #2="low limit") -> (element #1=w334:dbl[], element #2=w331:dbl[])  [unwired: 2 in]
            n167 = Array Max & Min(array=w336) -> (max value=w330:dbl)  [unwired: 3 out]
            n168 = Array Max & Min(array=w335) -> (max value=w329:dbl)  [unwired: 3 out]
            n169 = Array Max & Min(array=w334) -> (max value=w328:dbl)  [unwired: 3 out]
            n170 = Array Max & Min(array=w331) -> (max value=w327:dbl)  [unwired: 3 out]
            n171 = Wait Until Next ms Multiple(millisecond multiple="frame [ms]") -> ()  [unwired: 1 out]
            n172 = Less?(x=w330, y="thresh2") -> (x < y?=w322:bool)
            n173 = Less?(x=w329, y="thresh2") -> (x < y?=w323:bool)
            n174 = Less?(x=w328, y="thresh2") -> (x < y?=w324:bool)
            n175 = Less?(x=w327, y="thresh2") -> (x < y?=w325:bool)
            n176 = Compound Arithmetic op=AND(w322, w323, w324, w325) -> (w321:bool)
            "result" <- w321
            n177 = call "segmentation.vi"("unmixed ch2"=w313, "segmentation method"="seg meth 2", "image lpf"="lpf 2", "post processing"="post proc 2", "input cluster"="input 2", "Threshold Limits"="Threshold Limits 2") -> ("Array"=w350:u8[][])  [unwired: 7 in, 2 out]
            n178 = call "segmentation.vi"("unmixed ch2"=w314, "segmentation method"="seg meth", "image lpf"="lpf 1", "post processing"="post proc1", "input cluster"="in1", "Threshold Limits"="Threshold Limits") -> ("Array"=w351:u8[][])  [unwired: 7 in, 2 out]
            n179 = Add Array Elements(numeric array=w350) -> (sum=w349:u8)
            n180 = Less?(x="decline thresh", y=w317) -> (x < y?=w346:bool)
            "x < y?" <- w346
            n181 = Not Equal To 0?(x=w349) -> ()  [unwired: 1 out]
            n182 = Compound Arithmetic op=AND(w346, w321, w306) -> (w347:bool)
            n183 = Or(x=w347, y=w341) -> (x .or. y?=w342:bool)
            n184 = case shown="True" w342 {
              tunnel: w314 -> [_ w443]
              tunnel: w313 -> [_ w448]
              tunnel: w351 -> [_ w433]
              tunnel: w350 -> [_ w432]
              tunnel: w344 -> [_ w445]
              tunnel: w317 -> [_ w444]
              tunnel: w348 -> [w423 _]
              tunnel: w305 -> [_ w439]
              tunnel: w304 -> [_ w438]
              tunnel: w303 -> [_ w437]
              tunnel: w302 -> [_ w436]
              tunnel: w301 -> [_ w430]
              frame False {
                n185 = local read "frame index"() -> (w424:i32)
                n186 = case shown="True" w423 {
                  tunnel: w424 -> [w427 w429]
                  tunnel: [w426 w428] -> w425
                  frame False {
                    n187 = Decrement(x=w427) -> (x-1=w426:i32)
                  }
                  frame True {
                    n188 = Increment(x=w429) -> (x+1=w428:i32)
                  }
                }
                n189 = local write "frame index"(w425) -> ()
              }
              frame True {
                # "画像表示と設定"
                n190 = call "merge segmented areas.vi"("iterations (1)"="iter", "mergin array"="mgn", "Array"=w432, "Array 2"=w433) -> ("Array out"=w431:u8[][])  [unwired: 6 in, 1 out]
                n191 = local read "show imgs"() -> (w442:bool)
                n192 = local read "N of success"() -> (w441:u16)
                n193 = case shown="True" w442 {
                  tunnel: w443 -> [_ w458]
                  tunnel: w448 -> [_ w466]
                  tunnel: w431 -> [_ w462]
                  tunnel: w433 -> [_ w457]
                  tunnel: w432 -> [_ w465]
                  tunnel: w445 -> [_ w474]
                  tunnel: w444 -> [_ w473]
                  frame False {
                  }
                  frame True {
                    n194 = call "create histogram of masked image.vi"("Array in"=w462, "unmixed ch1"=w458, "intervals"="intervals") -> ("Histogram Graph"=→"Histogram":T2)  [unwired: 8 in]
                    n195 = call "extract outline by gradient out.vi"("input mask"=w462) -> ("Array out 2"=w469:u8[][])  [unwired: 1 in]
                    n196 = case shown="True" "autoscale" {
                      tunnel: w473 -> [_ w497]
                      tunnel: w474 -> [_ w496]
                      tunnel: "color" -> [w486 w493]
                      tunnel: [w486 w492] -> w472
                      frame False {
                      }
                      frame True {
                        n197 = Multiply(x=w497, y="scale fac1") -> (x*y=w491:dbl)
                        n198 = Index Array(array=w493) -> (element #1=w499:T3, element #2=w498:T3, element #3=w487:T3)  [unwired: 3 in]
                        n199 = Multiply(x=w496, y="scale fac2") -> (x*y=w490:dbl)
                        n200 = Bundle(cluster=w499, "max"=w491) -> (w495:T3)  [unwired: 3 in]
                        n201 = Bundle(cluster=w498, "max"=w490) -> (w494:T3)  [unwired: 3 in]
                        n202 = Build Array(w495, w494, w487) -> (w492:T8)
                      }
                    }
                    n203 = Array Size(array=w458) -> (size(s)=w475:i32[])
                    n204 = Multiply(x="zoom", y=w475) -> (x*y=w476:dbl[])
                    n205 = property on="ch1" class="Pict"("ZoomFactor"="zoom") -> ()  [unwired: 2 in, 2 out]
                    n206 = property on="ch2" class="Pict"("ZoomFactor"="zoom") -> ()  [unwired: 2 in, 2 out]
                    n207 = property on="mixed" class="Pict"("ZoomFactor"="zoom") -> ()  [unwired: 2 in, 2 out]
                    n208 = Index Array(array=w476) -> (element #1=w463:dbl, element #2=w464:dbl)  [unwired: 2 in]
                    n209 = Bundle By Name(cluster="Draw Area Size", "Width"=w463, "Height"=w464) -> (w479:T10)
                    n210 = property on="mask1" class="IntGraph (strict)"("Height"=w464, "Width"=w463) -> ()  [unwired: 2 in, 2 out]
                    n211 = Multiply(x=w458, y=w457) -> (x*y=w468:dbl[][])
                    n212 = Multiply(x=w466, y=w465) -> (x*y=w467:dbl[][])
                    n213 = property on="ch1" class="Pict"("Draw Area Size"=w479) -> ()  [unwired: 2 in, 2 out]
                    n214 = property on="ch2" class="Pict"("Draw Area Size"=w479) -> ()  [unwired: 2 in, 2 out]
                    n215 = property on="mixed" class="Pict"("Draw Area Size"=w479) -> ()  [unwired: 2 in, 2 out]
                    n216 = property on="mask2" class="IntGraph (strict)"("Height"=w464, "Width"=w463) -> ()  [unwired: 2 in, 2 out]
                    n217 = Select(t=w458, s="mask img", f=w468) -> (s? t:f=w459:dbl[][])
                    n218 = Select(t=w466, s="mask img", f=w467) -> (s? t:f=w481:dbl[][])
                    n219 = call "3color creation-cluster-2.vi"("color"=w472, "Array 4"=bool[] [TRUE, TRUE, TRUE], "Array 3"=w469, "Array 2"=w481, "Array"=w459) -> ("new picture"=→"mixed":picture, "ch2"=→"ch2":picture, "ch1"=→"ch1":picture)  [unwired: 1 in, 1 out]
                    "mask1" <- w457
                    "mask2" <- w465
                    "cs" <- w466
                    "cs 2" <- w458
                  }
                }
                n220 = Increment(x=w441) -> (x+1=w440:u16)
                n221 = local write "N of success"(w440) -> ()
                n222 = To Word Integer(number=w443) -> (16bit integer=w435:i16[][])
                n223 = To Word Integer(number=w448) -> (16bit integer=w434:i16[][])
                n224 = case shown="True" w430 {
                  tunnel: w439 -> [_ w456]
                  tunnel: w438 -> [_ w455]
                  tunnel: w437 -> [_ w454]
                  tunnel: w436 -> [_ w453]
                  tunnel: w435 -> [_ w452]
                  tunnel: w434 -> [_ w451]
                  tunnel: w433 -> [_ w450]
                  tunnel: w432 -> [_ w449]
                  frame False {
                  }
                  frame True {
                    n225 = Enqueue Element(queue=w455, element=w451) -> ()  [unwired: 2 in, 3 out]
                    n226 = Enqueue Element(queue=w454, element=w450) -> ()  [unwired: 2 in, 3 out]
                    n227 = Enqueue Element(queue=w453, element=w449) -> ()  [unwired: 2 in, 3 out]
                    n228 = Enqueue Element(queue=w456, element=w452) -> ()  [unwired: 2 in, 3 out]
                  }
                }
              }
            }
          }
        }
      }
      "curr index" <- w177
    }
    n229 = case shown="True" w37 {
      tunnel: w29 -> [w55 w79]
      tunnel: w28 -> [w54 w78]
      tunnel: w27 -> [w53 w77]
      tunnel: w26 -> [w52 w76]
      frame False {
        n230 = Release Queue(queue=w55) -> ()  [unwired: 2 in, 3 out]
        n231 = Release Queue(queue=w54) -> ()  [unwired: 2 in, 3 out]
        n232 = Release Queue(queue=w53) -> ()  [unwired: 2 in, 3 out]
        n233 = Release Queue(queue=w52) -> ()  [unwired: 2 in, 3 out]
        n234 = local write "stop"(FALSE) -> ()
      }
      frame True {
        w60 = "-" ("string")
        w84 = T12."replace or create" ("operation (0:open)")
        n235 = Get Queue Status(queue=w79) -> (# elements in queue=w80:i32)  [unwired: 2 in, 7 out]
        n236 = for {
          N: w80 -> [_]
          tunnel: w79 -> [w104]
          tunnel: w78 -> [w103]
          tunnel: w77 -> [w102]
          tunnel: w76 -> [w101]
          tunnel: [w100] -> w74 mode=indexing
          tunnel: [w99] -> w75 mode=indexing
          tunnel: [w98] -> w73 mode=indexing
          tunnel: [w97] -> w72 mode=indexing
          tunnel: [w96] -> w69
          tunnel: [w95] -> w68
          tunnel: [w94] -> w67
          tunnel: [w93] -> w66
          n237 = Dequeue Element(queue=w104) -> (queue out=w96:refnum<queue>, element=w99:i16[][])  [unwired: 2 in, 2 out]
          n238 = Dequeue Element(queue=w103) -> (queue out=w95:refnum<queue>, element=w100:i16[][])  [unwired: 2 in, 2 out]
          n239 = Dequeue Element(queue=w102) -> (queue out=w94:refnum<queue>, element=w98:u8[][])  [unwired: 2 in, 2 out]
          n240 = Dequeue Element(queue=w101) -> (queue out=w93:refnum<queue>, element=w97:u8[][])  [unwired: 2 in, 2 out]
        }
        n241 = Release Queue(queue=w69) -> ()  [unwired: 2 in, 3 out]
        n242 = Release Queue(queue=w68) -> ()  [unwired: 2 in, 3 out]
        n243 = Release Queue(queue=w67) -> ()  [unwired: 2 in, 3 out]
        n244 = Release Queue(queue=w66) -> ()  [unwired: 2 in, 3 out]
        n245 = local read "appended path"() -> (w56:path)
        n246 = Build Array(w75, w74) -> (w70:i16[][][][])
        n247 = Build Array(w73, w72) -> (w71:u8[][][][])
        n248 = Strip Path(path=w56) -> (stripped path=w83:path, name=w57:string)
        n249 = Search and Replace String(input string=w57, search string=".tif" ("substring (\"\")"), replace string=".FIRE" ("replace string (\"\")")) -> (result string=w59:string)  [unwired: 5 in, 3 out]
        n250 = Strip Path(path=w83) -> (stripped path=w82:path, name=w81:string)
        n251 = Search and Replace String(input string=w57, search string=".tif" ("substring (\"\")"), replace string="mask.FIRE" ("replace string (\"\")")) -> (result string=w58:string)  [unwired: 5 in, 3 out]
        n252 = local write "stop"(FALSE) -> ()
        n253 = Concatenate Strings(w81, w60, w59) -> (w88:string)
        n254 = Concatenate Strings(w81, w60, w58) -> (w87:string)
        n255 = Build Path(base path=w82, name or relative path=w88) -> (appended path=w86:path)
        n256 = Build Path(base path=w82, name or relative path=w87) -> (appended path=w85:path)
        n257 = Open/Create/Replace File(file path (use dialog)=w85, operation (0:open)=w84) -> (refnum out=w89:refnum<file>)  [unwired: 4 in, 2 out]
        n258 = Open/Create/Replace File(file path (use dialog)=w86, operation (0:open)=w84) -> (refnum out=w92:refnum<file>)  [unwired: 4 in, 2 out]
        n259 = Write to Binary File(file (use dialog)=w92, data=w70) -> (refnum out=w91:refnum<file>)  [unwired: 4 in, 2 out]
        n260 = Write to Binary File(file (use dialog)=w89, data=w71) -> (refnum out=w90:refnum<file>)  [unwired: 4 in, 2 out]
        n261 = Close File(refnum=w91) -> ()  [unwired: 1 in, 2 out]
        n262 = Close File(refnum=w90) -> ()  [unwired: 1 in, 2 out]
      }
    }
    "N of success" <- u16 0
    "appended path" <- w25
    "current file index" <- w22
  }
